vi "FID Scan.vi"(6 "Purpose":string, 8 "error in (no error)":errorcluster) -> (0 "error out":errorcluster, 1 "Cancel ?":bool, 3 "data":T1)   [LabVIEW 2020]
uses:
  Controls/1775E_Authen_Level.ctl
  Controls/user_log.ctl
  <vilib>/Utility/miscctls.llb/LVPointTypeDef.ctl
  Controls/User_DB.ctl
  <vilib>/Instr/_visa.llb/VISA Configure Serial Port (Instr).vi
  <vilib>/addons/database/Connection.llb/Conn Execute.vi
  <vilib>/addons/database/Recordset.llb/Rec Fetch Recordset Data (R).vi
  691E_Global.vi
  <vilib>/addons/database/Recordset.llb/Rec Destroy - Connection.vi
  <vilib>/addons/database/NI_Database_API.lvlib
panel:
  out "Cmd Suceed?":bool
  in  "Hide":bool
  out "Device Info":string
  out "Array":string[](array[string])
  out "State":string
  out "Numeric":i32
  in  "Password":string
  in  "Cancel":bool
  in  "Ok":bool
  in  "View Log":bool
  out "Cmd.":bool
  in  "Super User":bool
  in  "View All":bool
  out "String":string
  in  "Clock No.":string(combo)
  in  "Level":T2
  in  "User Name":string(combo)
  in  "ID Number":i16
  out "Finger Present?":bool
  out "Response":string
  in  "Delete All":bool
  in  "Delete":bool
  in  "Search":bool
  in  "Enroll":bool
  out "Status":string
  out "elements":u8[](array[numeric]) format="%.0x"
  in  "Stop":bool
  out "Buffer Out":string
  in  "write buffer":string="ï\u0001ÿÿÿÿ\u0001\u0000\u00034\u00008"
  out "Profile Image":picture
  # "User Access Login"
  # "thumb finger"
  # "EF01 FFFF FFFF 0700 0700 0003 00A4 00B5"
  # "EF01 FFFF FFFF 0700 0709 0003 0028 0042"
  # "EF01 FFFF FFFF 0700 0700 0000 0065 0073"
  # "EF01 FFFF FFFF 0700 0700 0001 0084 0093"
  # "EF01 FFFF FFFF 0700 0709 0003 0002 001C"
  # "wrong finger"
  # "EF01 FFFF FFFF 0700 0703 0000 0000 0011"
  # "NO finger"
  # "EF01 FFFF FFFF 0700 0703 0000 0000 0011"
  # "EF01 FFFF FFFF 0700 0703 0000 0000 0011"
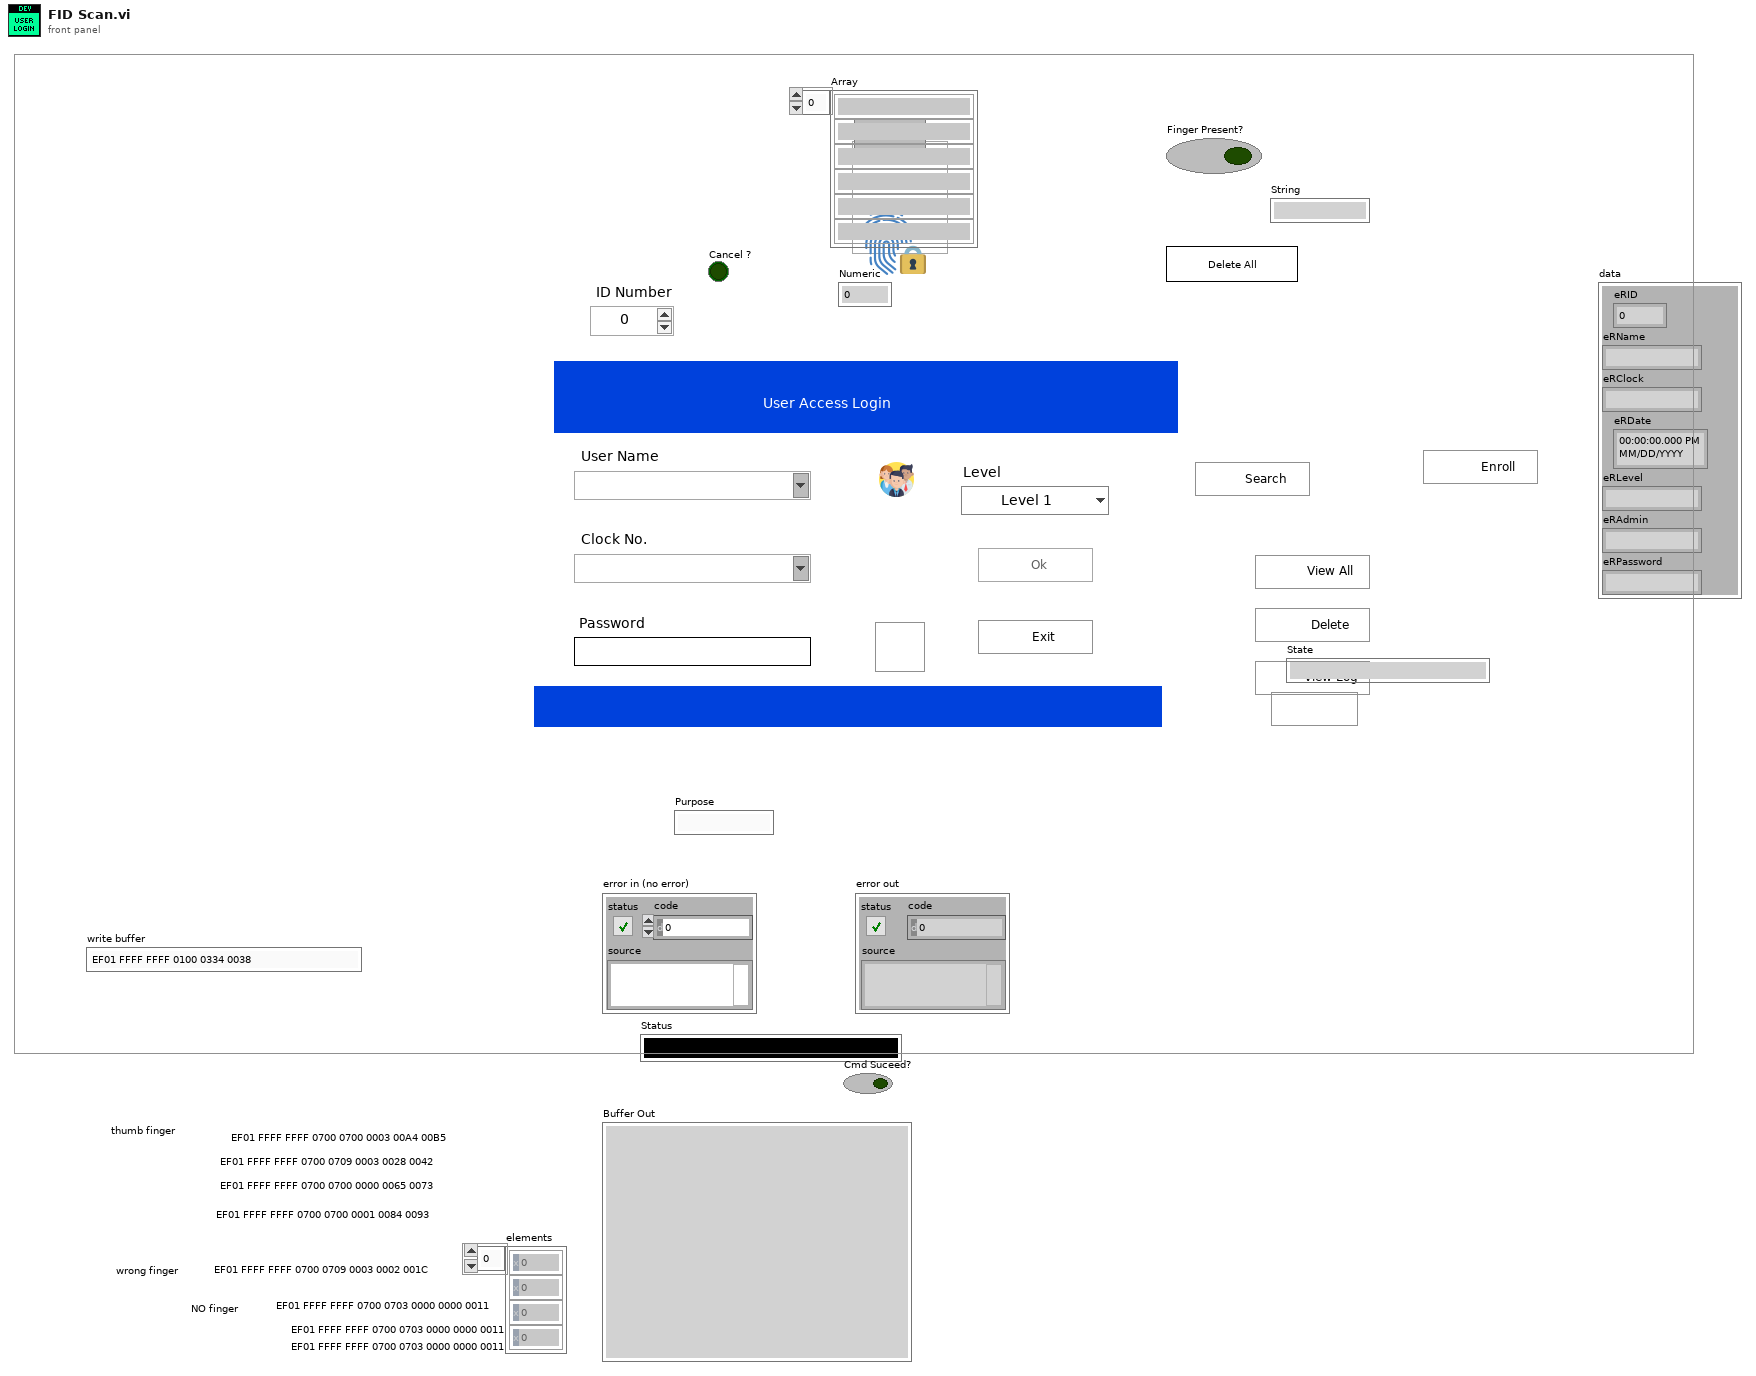
[diagram p1: front panel]
types:
  T1 = typedef "user_log.ctl" = cluster{"eRID":u16, "eRName":string, "eRClock":string, "eRDate":timestamp, "eRLevel":string, "eRAdmin":string, "eRPassword":string}
  T2 = typedef "1775E_Authen_Level.ctl" = enum16{"Level 1", "Level 2", "Level 3", "Level 4", "Super Level"}
  T3 = typedef "LVPointTypeDef.ctl" = cluster{"Horizontal":i16, "Vertical":i16}
  T4 = enum8{"Enabled", "Disabled", "Disabled and Grayed Out"}
  T5 = typedef "TD SQL.ctl" = cluster{"MS SQL Connection":T6, "UDL File":path, "Time":string, "DCODE":string, "WIP+1":i64, "MC No?":i32, "POKAYOKE?":bool, "Expected Result":string, "Result [Status]":string, "Clock":dbl, "RFID":string, "WIP Queue":refnum<queue>, "TS Parameter":T7, "Data_Queue":refnum<queue>[], "RFID Serial No.":string}
  T6 = typedef "NI_Database_API.lvlib/Conn ObjectReference.ctl" = refnum<k1>
  T7 = typedef "TS_Parameter.ctl" = cluster{"ProfitCenterCode":string, "LineCode":string, "WorkOrderNumber":string, "Model":string, "Model_with_Prefix":string, "VendorCode":string, "SetParameterDateCode":string, "PokaYoke":i32, "Target":i32, "Live_DateCode":string, "CustomerPartNumber":string, "Hand":string, "sBarcode":bool, "FCA":i32, "Ent_Stamp":timestamp, "STS_CD":dbl}
  T8 = typedef "User_DB.ctl" = cluster{"eRID":u16, "eRName":string, "eRClock":string, "eRDate":timestamp, "eRLevel":string, "eRAdmin":string, "eRPassword":string, "eRPurpose":string}
  T9 = typedef "NI_Database_API.lvlib/Rec ObjectReference.ctl" = refnum<k1>
  T10 = typedef "LVBoundsTypeDef.ctl" = cluster{"Width":u32, "Height":u32}
  T11 = typedef "imagedata.ctl" = cluster{"image type":i32, "image depth":i32, "image":u8[], "mask":u8[], "colors":u32[], "Rectangle":cluster{"left":i16, "top":i16, "right":i16, "bottom":i16}}
  T12 = cluster{"left":i16, "top":i16, "right":i16, "bottom":i16}
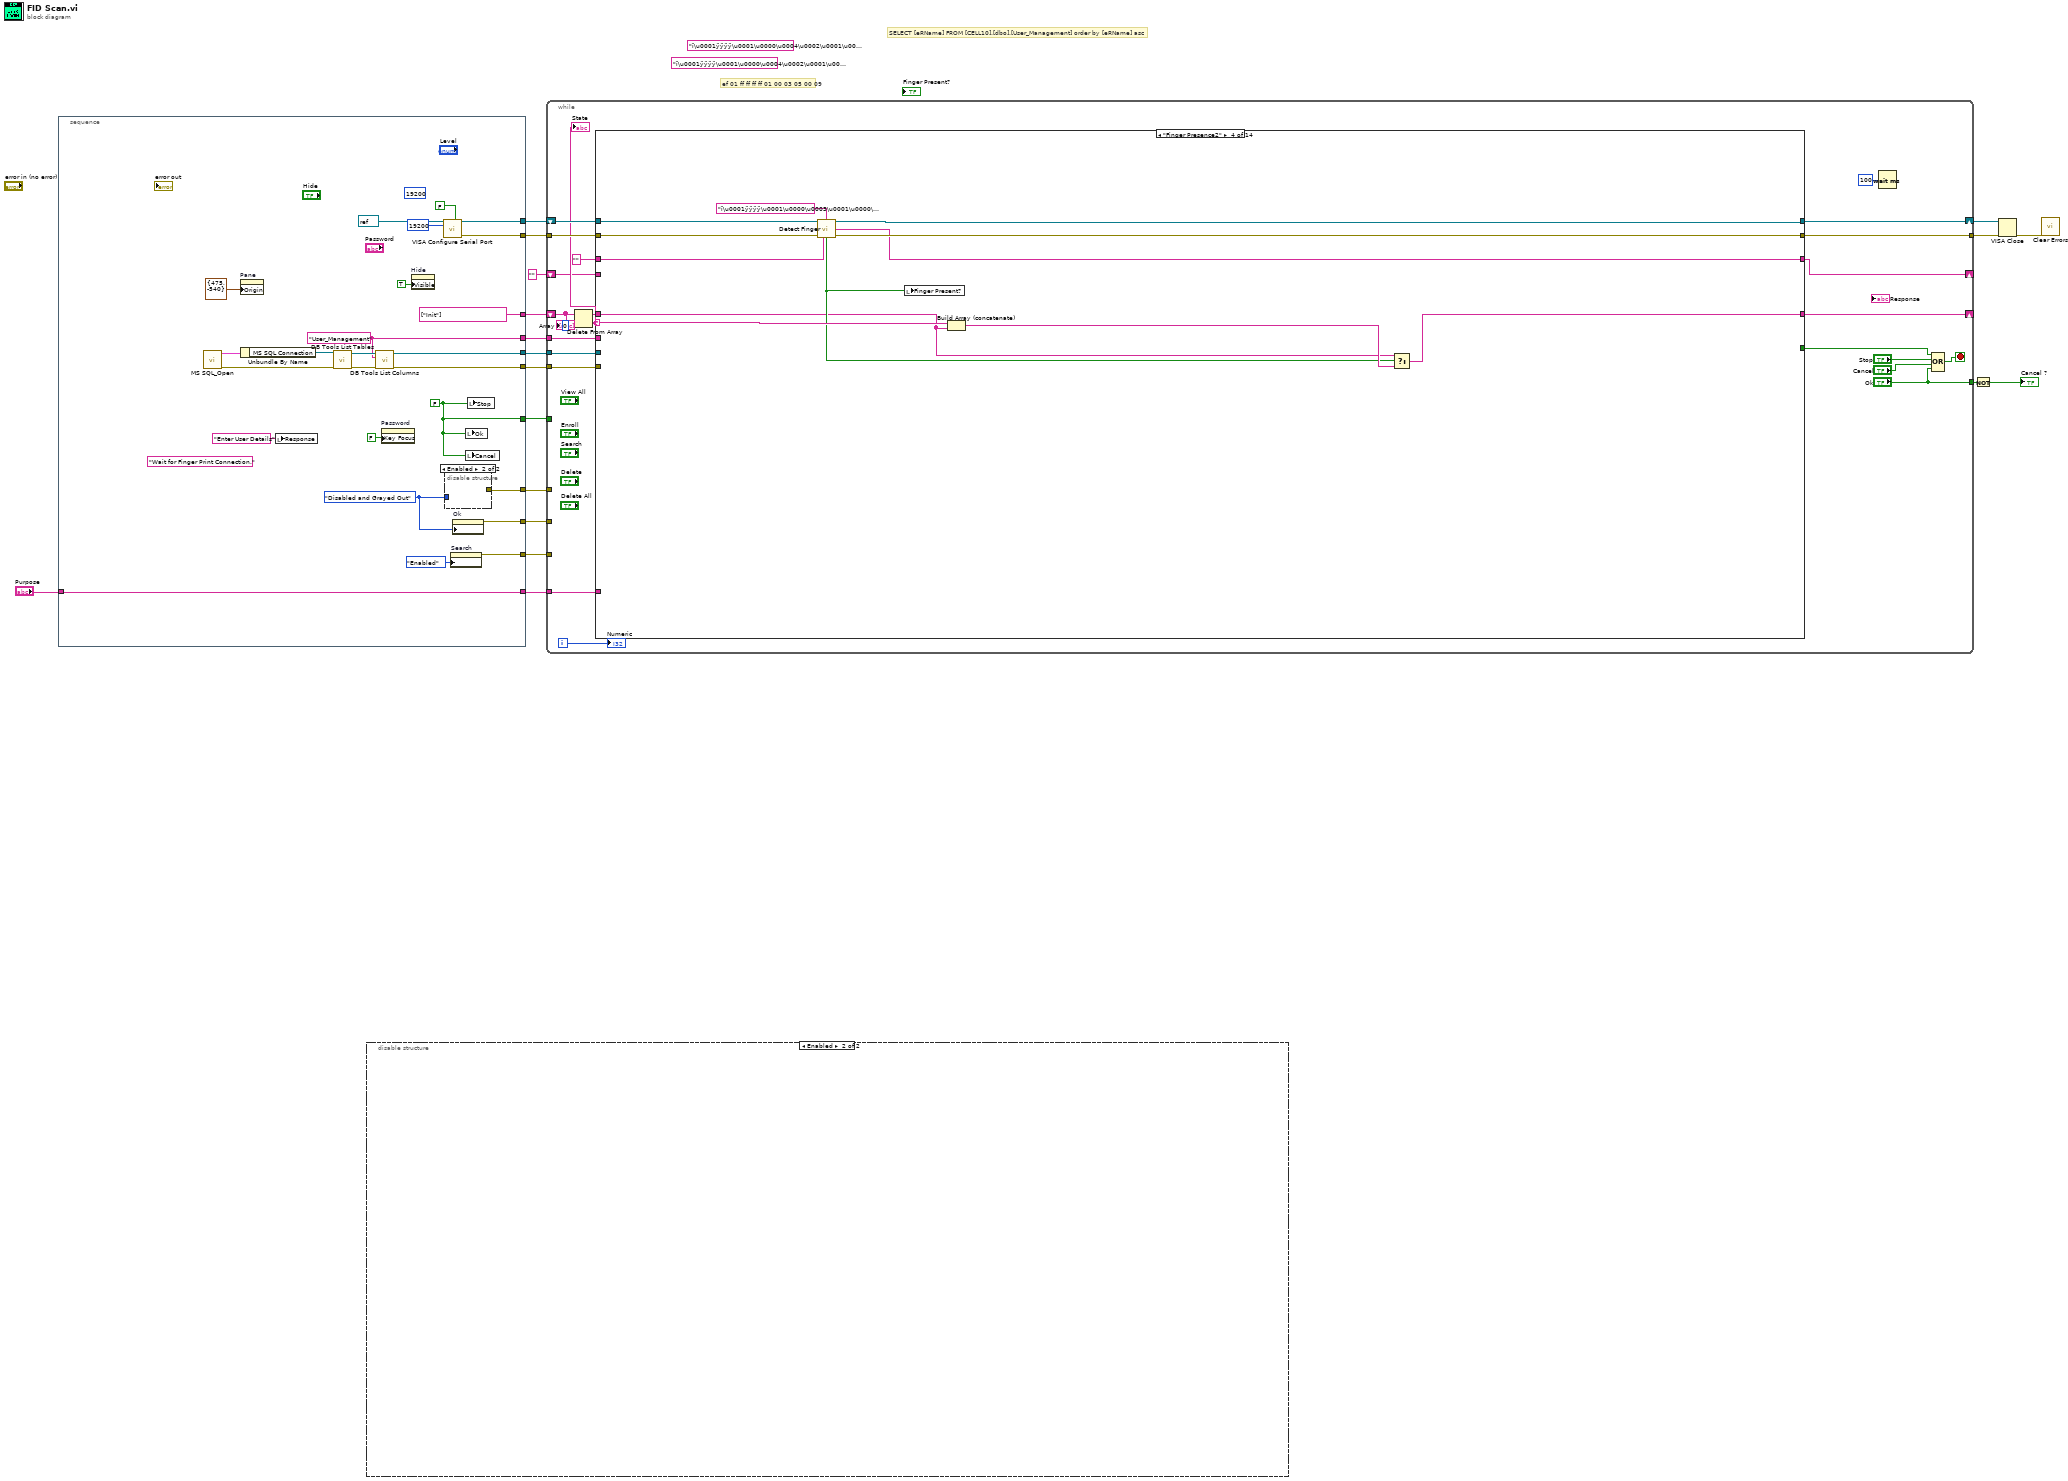
[diagram p0: block diagram]
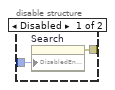
[diagram p2: hidden frame]
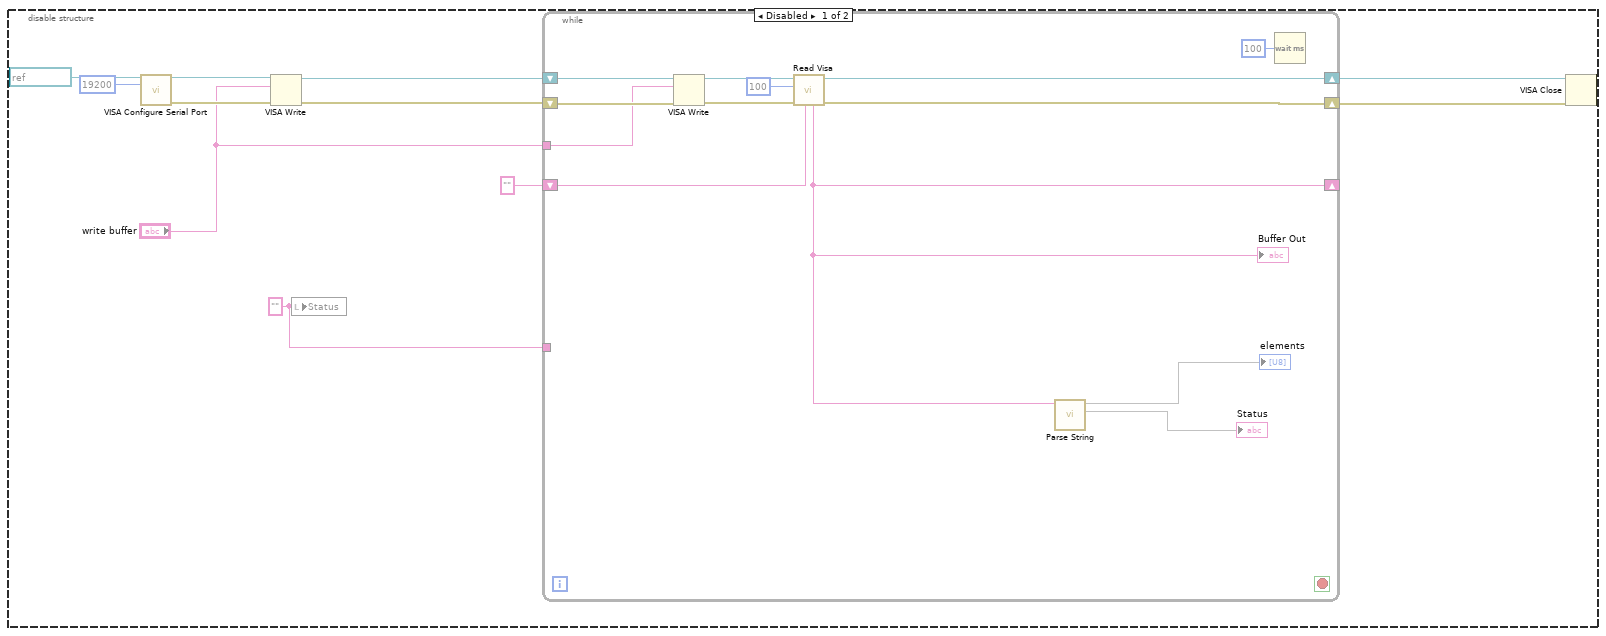
[diagram p3: hidden frame]
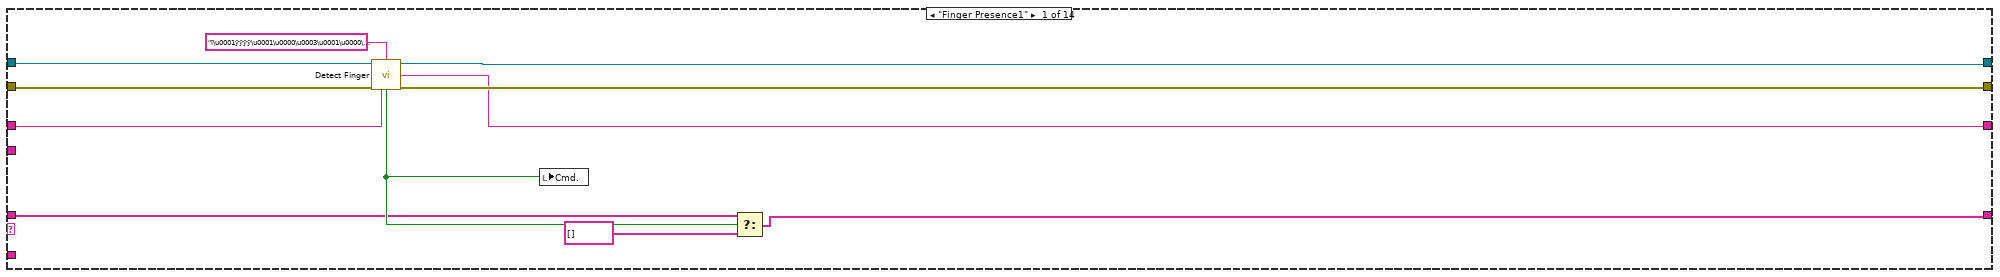
[diagram p4: hidden frame]
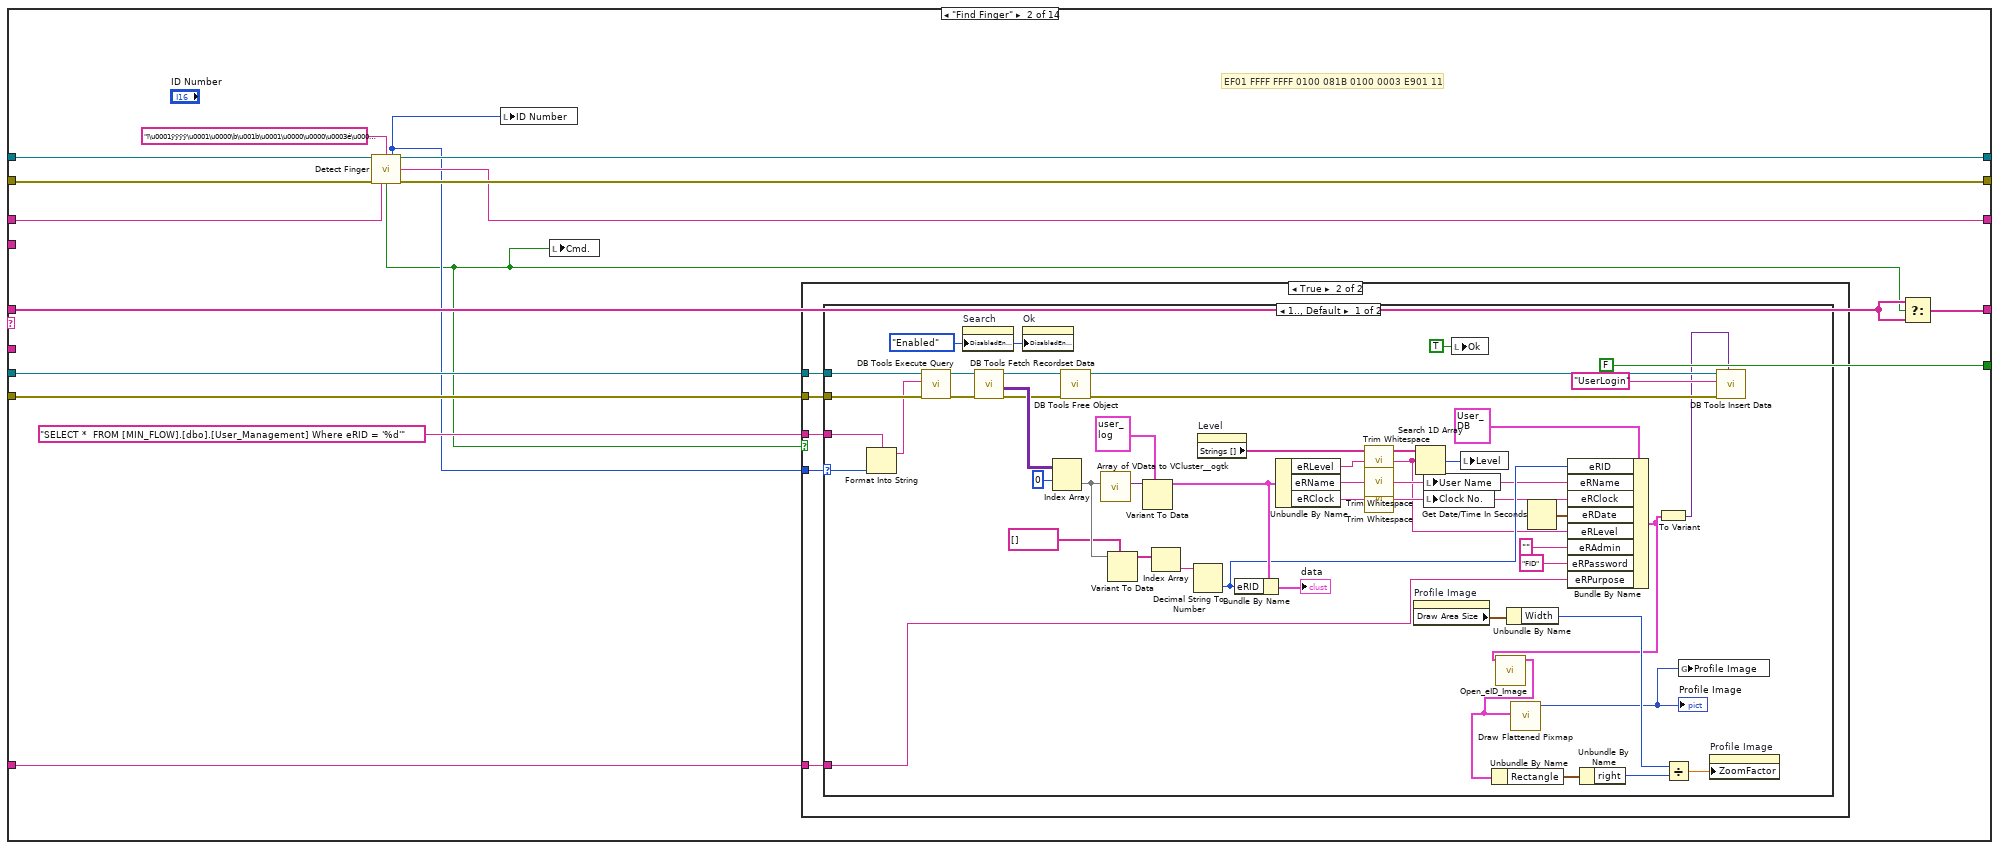
[diagram p5: hidden frame]
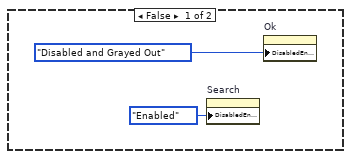
[diagram p6: hidden frame]
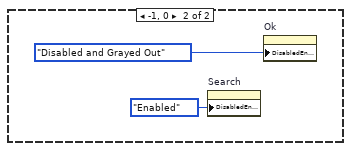
[diagram p7: hidden frame]
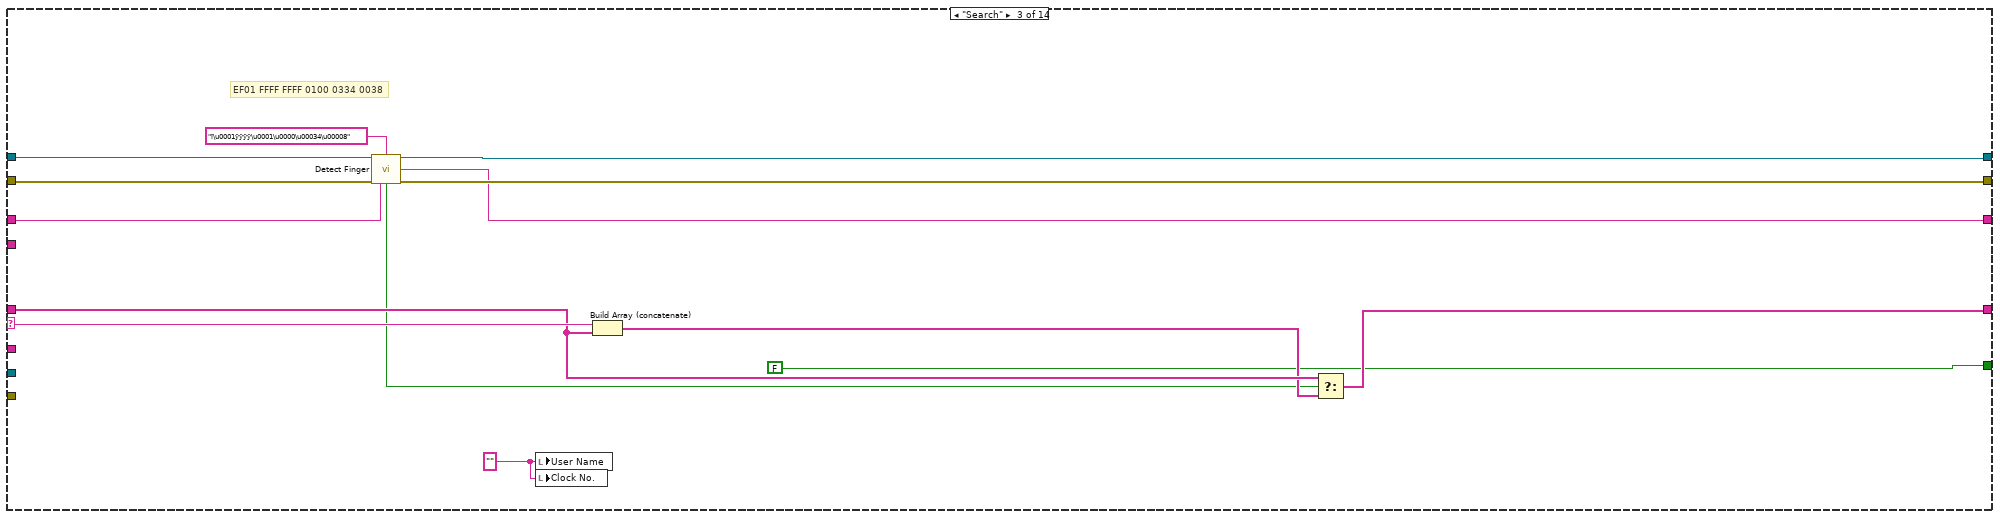
[diagram p8: hidden frame]
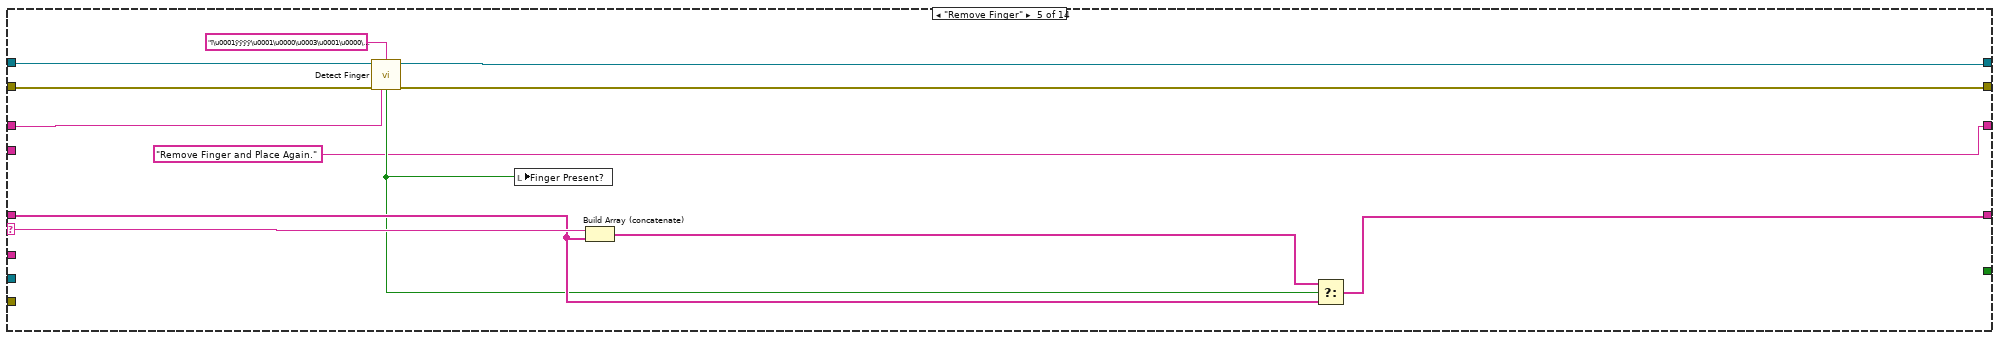
[diagram p9: hidden frame]
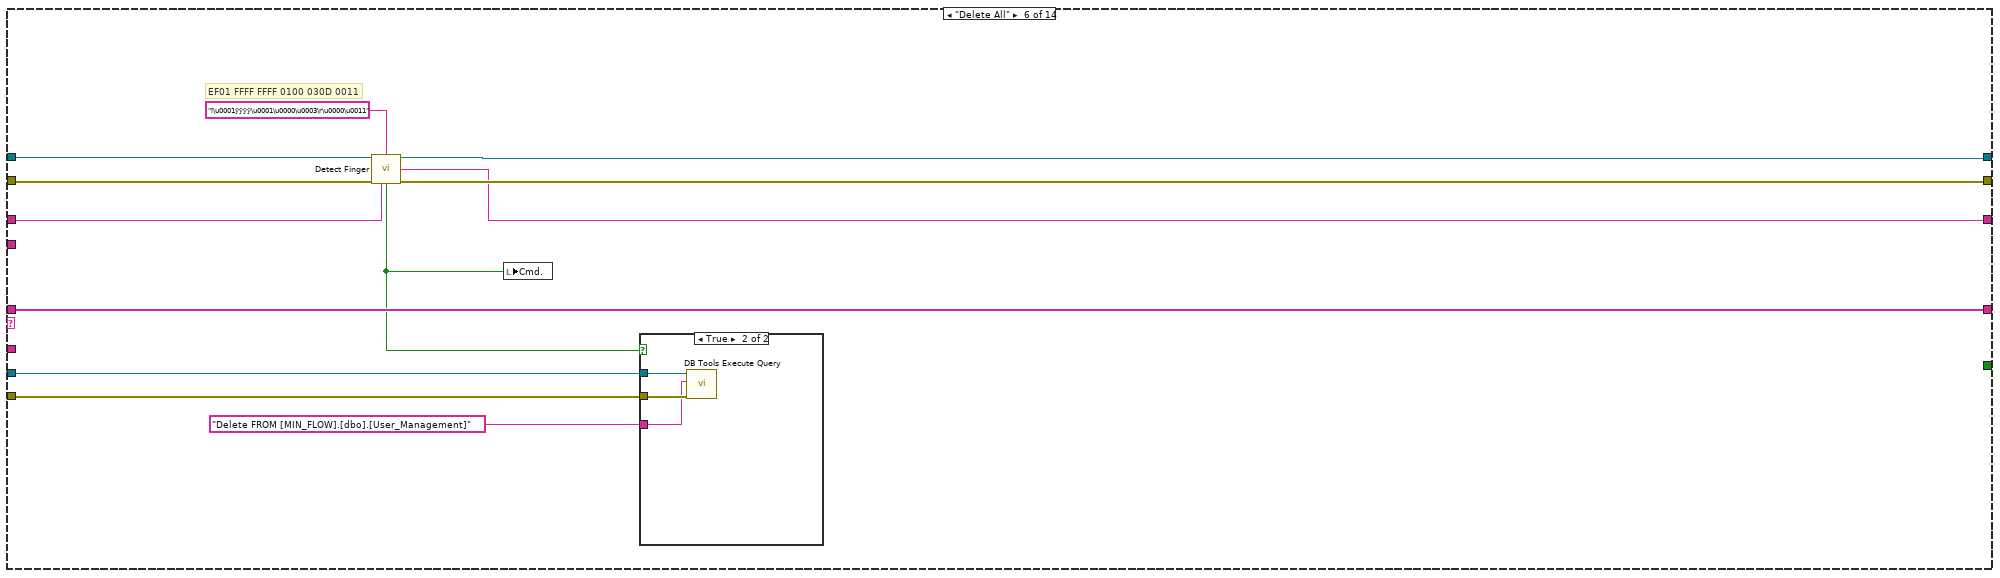
[diagram p10: hidden frame]
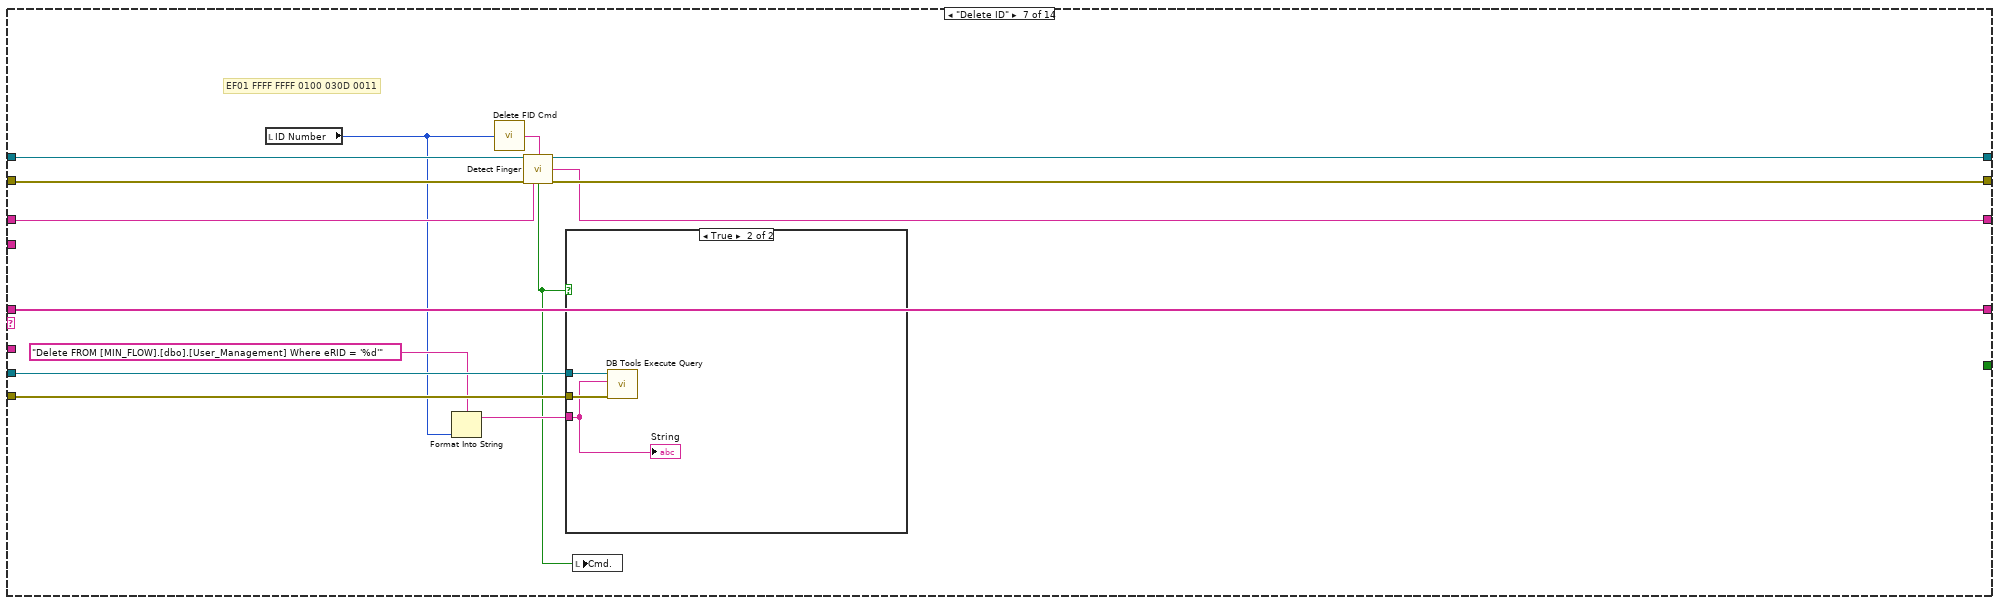
[diagram p12: hidden frame]
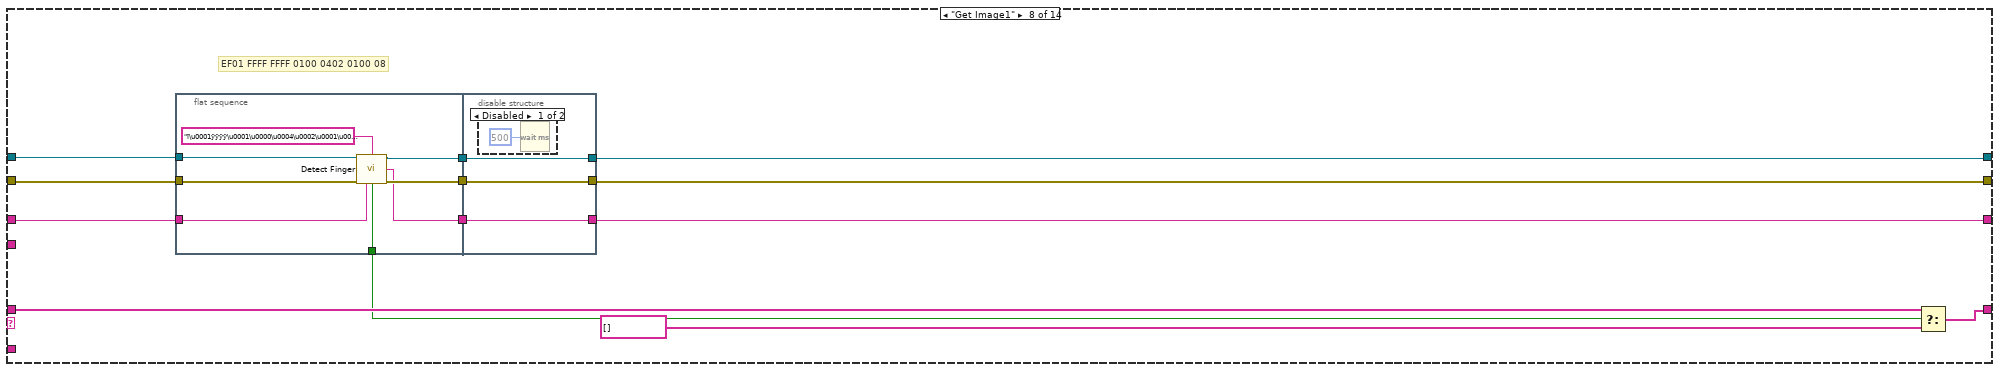
[diagram p14: hidden frame]
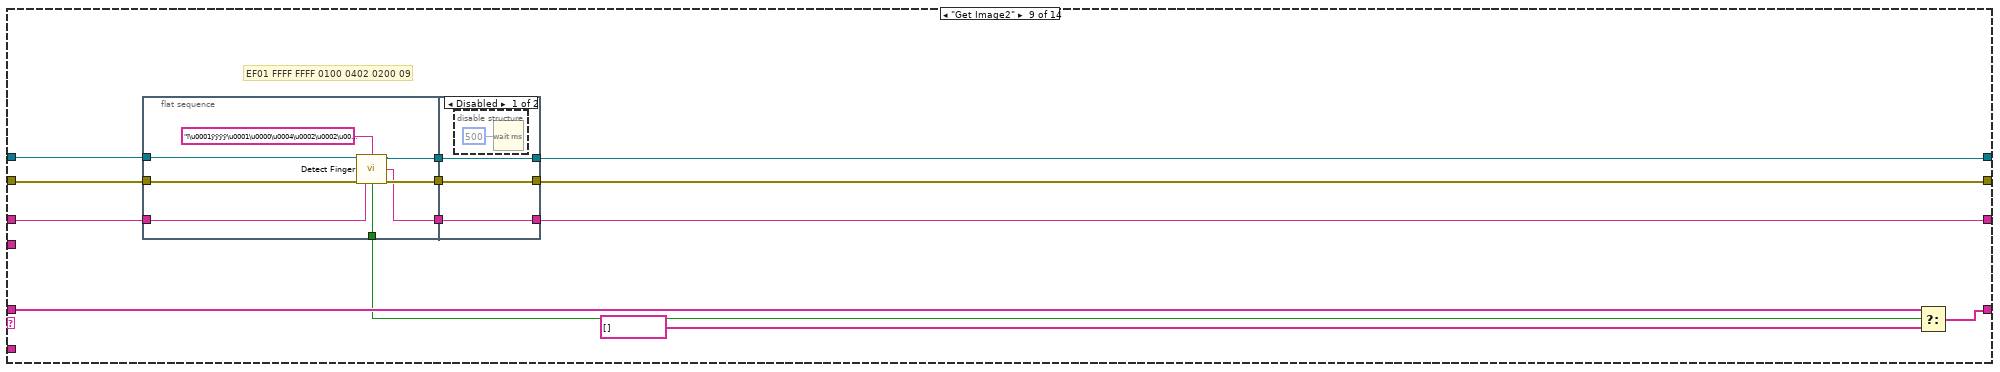
[diagram p16: hidden frame]
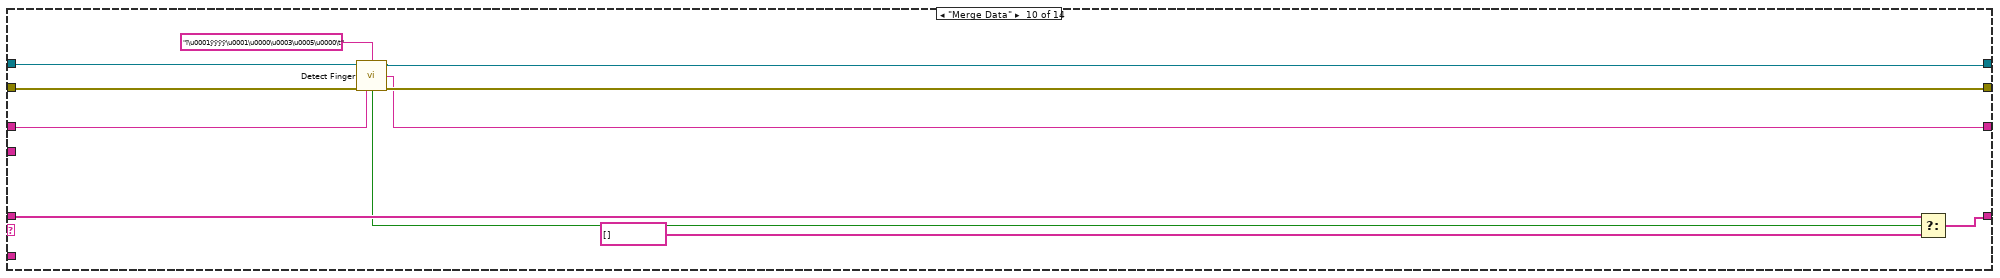
[diagram p18: hidden frame]
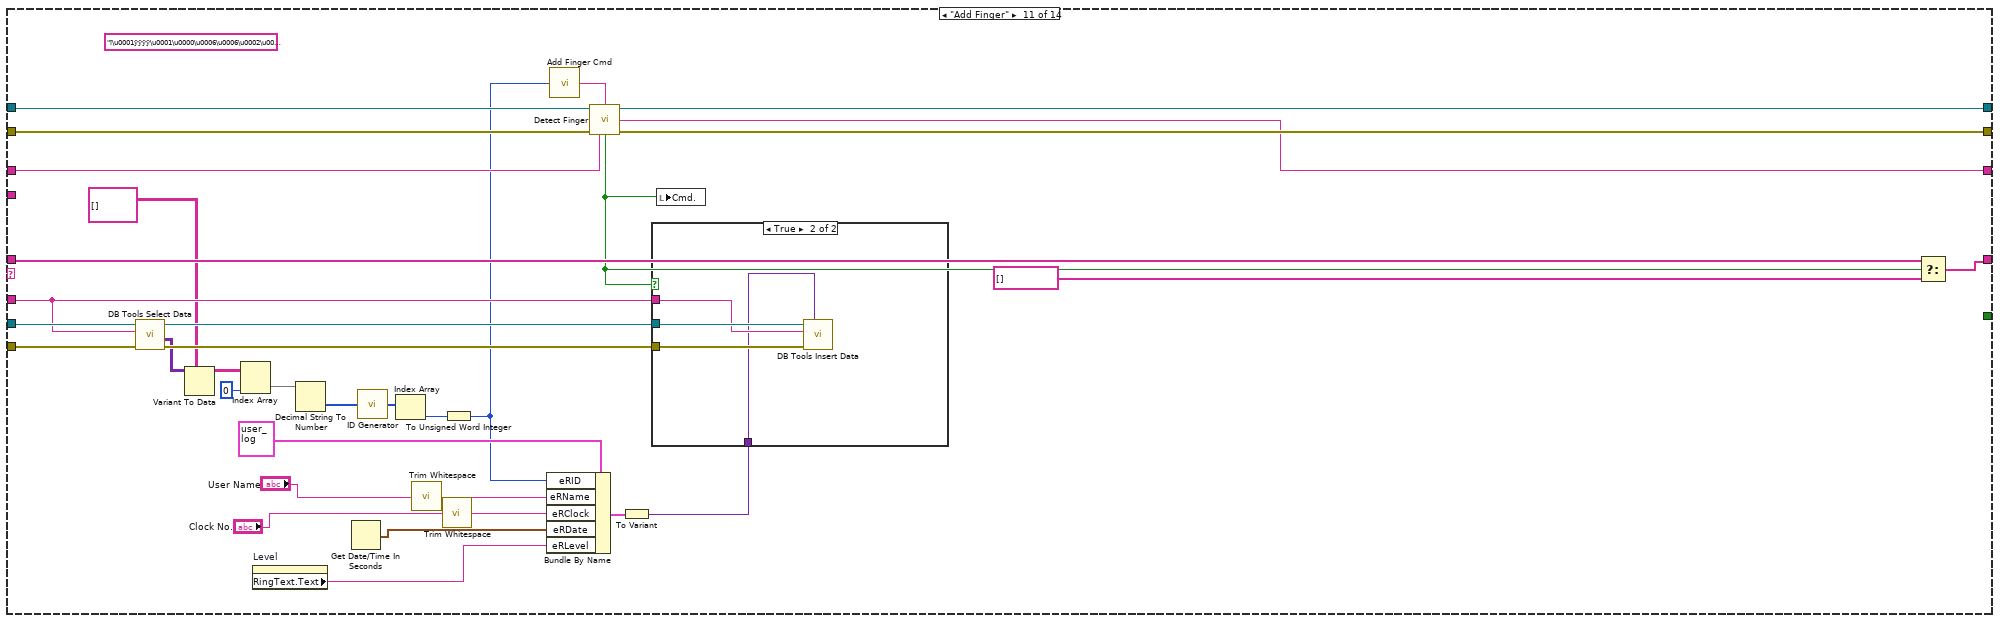
[diagram p19: hidden frame]
diagram:
  (unwired) "ï\u0001ÿÿÿÿ\u0001\u0000\u0004\u0002\u0001\u0000\b" ("write buffer")
  (unwired) "ï\u0001ÿÿÿÿ\u0001\u0000\u0004\u0002\u0001\u0000\b" ("write buffer")
  # "SELECT [eRName] FROM [CELL10].[dbo].[User_Management] order by [eRName] asc"
  # "ef 01 ff ff ff ff 01 00 03 05 00 09"
  n1 = stacked-sequence {
    tunnel: [string[] ["Init"]] -> w18
    tunnel: [w41] -> w17
    tunnel: [w40] -> w16
    tunnel: [w37] -> w11
    tunnel: [w36] -> w10
    tunnel: [w35] -> w9
    tunnel: [w34] -> w6
    tunnel: [w32] -> w5
    tunnel: [w31] -> w4
    tunnel: [w29] -> w3
    tunnel: [w20] -> w2
    tunnel: "Purpose" -> [w20]
    frame #0 {
      (unwired) "Wait for Finger Print Connection." ("Response")
      (unwired) u32 19200 ("baud rate (9600)")
      w33 = T4."Disabled and Grayed Out" ("Disabled")
      w34 = FALSE ("Stop")
      w35 = "User_Management" ("table")
      n2 = call "MS SQL_Open.vi"() -> ("error out"=w21:errorcluster, "Ref Out"=w23:T5)  [unwired: 9 in, 1 out]
      n3 = property on="Pane" class="Pane"("Origin"=T3 {"Horizontal"=475, "Vertical"=-540}) -> ()  [unwired: 2 in, 2 out]
      n4 = Unbundle By Name(w23) -> ("MS SQL Connection"=w22:T6)
      n5 = local write "Response"("Enter User Details" ("Response")) -> ()
      n6 = call <vilib>:"DB Tools List Tables.vi"("error in (no error)"=w21, "connection reference"=w22) -> ("error out"=w38:errorcluster, "connection reference out"=w39:T6)  [unwired: 3 in, 1 out]
      n7 = call <vilib>:"DB Tools List Columns.vi"("error in (no error)"=w38, "table"=w35, "connection reference"=w39) -> ("error out"=w36:errorcluster, "connection reference out"=w37:T6)  [unwired: 1 in, 2 out]
      n8 = property on="Password" class="Str"("Key Focus"=FALSE) -> ()  [unwired: 2 in, 2 out]
      n9 = property on="Hide" class="Bool"("Visible"=TRUE) -> ()  [unwired: 2 in, 2 out]
      n10 = call-poly "VISA Configure Serial Port"("VISA resource name"=refnum<visa-resource-name> refnum ("FID_Comm"), "Enable Termination\nChar (T)"=FALSE ("Enable Termination\nChar (T)"), "baud rate (9600)"=u32 19200) -> ("VISA resource name out"=w41:refnum<visa-resource-name>, "error out"=w40:errorcluster)  [unwired: 11 in]
      n11 = disable-structure shown="Enabled" {
        disable-tunnel: w33 -> [w45 _]
        disable-tunnel: [w44 _] -> w32
        frame Disabled {
          n12 = property on="Search" class="Bool (strict)"("DisabledEnum"=w45) -> (error out=w44:errorcluster)  [unwired: 2 in, 1 out]
        }
        frame Enabled {
        }
      }
      n13 = property on="Search" class="Bool (strict)"("DisabledEnum"=T4."Enabled" ("Disabled")) -> (error out=w29:errorcluster)  [unwired: 2 in, 1 out]
      n14 = property on="Ok" class="Bool (strict)"("DisabledEnum"=w33) -> (error out=w31:errorcluster)  [unwired: 2 in, 1 out]
      n15 = local write "Ok"(w34) -> ()
      n16 = local write "Cancel"(w34) -> ()
      n17 = local write "Stop"(w34) -> ()
    }
  }
  n18 = disable-structure shown="Enabled" {
    frame Disabled {
      w46 = "" ("Status")
      n19 = call-poly "VISA Configure Serial Port"("VISA resource name"=refnum<visa-resource-name> "COM6", "baud rate (9600)"=u32 19200) -> ("VISA resource name out"=w52:refnum<visa-resource-name>, "error out"=w50:errorcluster)  [unwired: 12 in]
      n20 = VISA Write(VISA resource name=w52, write buffer="write buffer", error in (no error)=w50) -> (VISA resource name out=w51:refnum<visa-resource-name>, error out=w49:errorcluster)  [unwired: 1 out]
      n21 = local write "Status"(w46) -> ()
      n22 = while {
        shift-right: [w70] -> w54
        shift-left: w51 -> [w64]
        shift-right: [w69] -> w53
        shift-left: w49 -> [w63]
        shift-right: [w59] -> _
        shift-left: "" ("Buffer Out") -> [w65]
        tunnel: "write buffer" -> [w60]
        tunnel: w46 -> [_]
        stop <- w67 stop-if-true
        n23 = VISA Write(VISA resource name=w64, write buffer=w60, error in (no error)=w63) -> (VISA resource name out=w61:refnum<visa-resource-name>, error out=w62:errorcluster)  [unwired: 1 out]
        n24 = call <userlib>:"Read Visa.vi"("Buffer In"=w65, "error in (no error)"=w62, "delay before read (ms)"=u32 100, "VISA Refnum in"=w61) -> ("error out"=w69:errorcluster, "VISA Refnum out"=w70:refnum<visa-resource-name>, "Buffer Out"=w59:string)  [unwired: 5 in]
        "Buffer Out" <- w59
        n25 = call "Parse String.vi"("Ack package"=w59) -> (2:→"Status", 3:→"elements")  [unwired: 7 in, 2 out]
        n26 = Wait (ms)(milliseconds to wait=u32 100) -> ()  [unwired: 1 out]
      }
      n27 = VISA Close(VISA resource name=w54, error in (no error)=w53) -> ()  [unwired: 1 out]
    }
    frame Enabled {
    }
  }
  n28 = while {
    shift-right: [w92] -> _
    shift-left: w18 -> [w93]
    tunnel: w16 -> [w90]
    shift-right: [w89] -> w14
    shift-left: w17 -> [w91]
    shift-right: [w79] -> _
    shift-left: "" ("Buffer Out") -> [w80]
    tunnel: [w86] -> w13
    tunnel: w11 -> [w78]
    tunnel: w10 -> [w77]
    tunnel: w9 -> [w76]
    tunnel: w6 -> [_]
    tunnel: ["Ok"] -> w8
    tunnel: w5 -> [_]
    tunnel: w4 -> [_]
    tunnel: w3 -> [_]
    tunnel: w2 -> [w71]
    i -> [w73]
    stop <- w84 stop-if-true
    n29 = Delete From Array(array=w93, index=0) -> (deleted portion=w83:string, array with subset deleted=w87:string[])  [unwired: 1 in]
    "State" <- w83
    n30 = case shown="\"Finger Presence2\"" w83 {
      selector: w83 -> [_ _ w190 w202 w214 _ _ _ _ _ _ _ _ _]
      tunnel: w87 -> [w95 w111 w189 w192 w213 w219 w236 w259 w284 w307 w341 w346 w360 w646]
      tunnel: [w94 w120 w187 w191 w211 w219 w236 w258 w283 w306 w340 w346 w359 w646] -> w92
      tunnel: w91 -> [w104 w119 w186 w200 w210 w226 w243 w256 w281 w304 w338 w349 w358 w644]
      tunnel: w90 -> [w103 w118 w185 w199 w209 w225 w242 w255 w280 w303 w337 w348 w357 w641]
      tunnel: [w101 w116 w183 w197 w207 w223 w240 w254 w279 w302 w336 w349 w356 w643] -> w89
      tunnel: [w102 w117 w184 w198 w208 w224 w241 w253 w278 w301 w335 w348 w355 w640] -> w86
      tunnel: [w100 w115 w182 w196 "Remove Finger and Place Again." ("Response") w222 w239 w251 w276 w299 w334 w347 w354 w645] -> w79
      tunnel: "" ("Buffer Out") -> [w97 w113 w178 w193 w204 w220 w238 w247 w272 w297 w332 w347 _ w642]
      tunnel: [_ FALSE ("Stop") FALSE ("Stop") _ _ _ _ _ _ _ _ _ _ _] -> w82
      tunnel: w80 -> [_ _ _ _ _ _ _ _ _ _ _ _ w354 _]
      tunnel: w78 -> [_ w110 _ _ _ w218 w235 _ _ _ w331 _ w353 w636]
      tunnel: w77 -> [_ w109 _ _ _ w217 w234 _ _ _ w330 _ w352 _]
      tunnel: w76 -> [_ _ _ _ _ _ _ _ _ _ w326 _ w351 _]
      tunnel: w71 -> [_ w105 _ _ _ _ _ _ _ _ _ _ w350 _]
      frame "Finger Presence1" {
        n31 = call "Detect Finger.vi"("VISA Refnum in"=w104, "Cmd"="ï\u0001ÿÿÿÿ\u0001\u0000\u0003\u0001\u0000\u0005" ("write buffer"), "error in (no error)"=w103, "Buffer In"=w97) -> ("VISA Refnum out"=w101:refnum<visa-resource-name>, "Response"=w100:string, "Cmd Suceed?"=w98:bool, "error out"=w102:errorcluster)  [unwired: 6 in, 2 out]
        n32 = local write "Cmd."(w98) -> ()
        n33 = Select(t=w95, s=w98, f=string[] []) -> (s? t:f=w94:string[])
      }
      frame "Find Finger" {
        # "EF01 FFFF FFFF 0100 081B 0100 0003 E901 11"
        n34 = call "Detect Finger.vi"("VISA Refnum in"=w119, "Cmd"="ï\u0001ÿÿÿÿ\u0001\u0000\b\u001b\u0001\u0000\u0000\u0003é\u0001\u0011" ("write buffer"), "error in (no error)"=w118, "Buffer In"=w113) -> ("ID"=w107:i16, "VISA Refnum out"=w116:refnum<visa-resource-name>, "Response"=w115:string, "Cmd Suceed?"=w106:bool, "error out"=w117:errorcluster)  [unwired: 6 in, 1 out]
        n35 = local write "ID Number"(w107) -> ()
        n36 = local write "Cmd."(w106) -> ()
        n37 = case shown="True" w106 {
          tunnel: w110 -> [_ w127]
          tunnel: w109 -> [_ w126]
          tunnel: "SELECT *  FROM [MIN_FLOW].[dbo].[User_Management] Where eRID = '%d'" ("SQL query") -> [_ w125]
          tunnel: w107 -> [_ w124]
          tunnel: w105 -> [_ w123]
          frame False {
            n38 = property on="Search" class="Bool (strict)"("DisabledEnum"=T4."Enabled" ("Disabled")) -> ()  [unwired: 2 in, 2 out]
            n39 = property on="Ok" class="Bool (strict)"("DisabledEnum"=T4."Disabled and Grayed Out" ("Disabled")) -> ()  [unwired: 2 in, 2 out]
          }
          frame True {
            n40 = case shown="1.., Default" w124 {
              selector: w124 -> [w171 _]
              tunnel: w127 -> [w153 _]
              tunnel: w126 -> [w173 _]
              tunnel: w125 -> [w172 _]
              tunnel: w123 -> [w128 _]
              frame 1.., Default {
                w140 = T4."Enabled" ("Disabled")
                n41 = Format Into String(format string=w172, w171) -> (resulting string=w170:string)  [unwired: 2 in, 1 out]
                n42 = call-poly <vilib>:"DB Tools Execute Query.vi"("error in (no error)"=w173, "SQL query"=w170, "connection reference"=w153) -> ("error out"=w174:errorcluster, "recordset reference"=w154:T9)  [unwired: 5 in]
                n43 = property on="Search" class="Bool (strict)"("DisabledEnum"=w140) -> ()  [unwired: 2 in, 2 out]
                n44 = call-poly <vilib>:"DB Tools Fetch Recordset Data.vi"("error in (no error)"=w174, "recordset reference"=w154) -> ("error out"=w150:errorcluster, "recordset data"=w166:variant[][], "recordset reference out"=w152:T9)  [unwired: 3 in]
                n45 = property on="Ok" class="Bool (strict)"("DisabledEnum"=w140) -> ()  [unwired: 2 in, 2 out]
                n46 = Index Array(array=w166, index (row)=0 ("disabled index (col)")) -> (element=w165:variant[])  [unwired: 1 in]
                n47 = call-poly <vilib>:"DB Tools Free Object.vi"("error in (no error)"=w150, "recordset reference"=w152) -> ("error out"=w149:errorcluster, "connection reference"=w151:T6)  [unwired: 8 in]
                n48 = call <userlib>:"Array of VData to VCluster__ogtk.vi"("Array"=w165) -> ("VCluster"=w168:variant)  [unwired: 9 in, 1 out]
                n49 = Variant To Data(type=string[] [], Variant=w165) -> (data=w163:string[])  [unwired: 1 in, 1 out]
                n50 = Variant To Data(type=T1 {"eRID"=0, "eRName"="", "eRClock"="", "eRDate"=timestamp(0 s since 1904-01-01), "eRLevel"="", "eRAdmin"="", "eRPassword"=""} ("Cluster"), Variant=w168) -> (data=w160:T1)  [unwired: 1 in, 1 out]
                n51 = Index Array(array=w163) -> (element=w162:string)  [unwired: 1 in]
                n52 = Decimal String To Number(string=w162) -> (number=w146:i32)  [unwired: 2 in, 1 out]
                n53 = property on="Level" class="Enum (strict)"() -> ("Strings []"=w155:string[])  [unwired: 2 in, 2 out]
                n54 = Bundle By Name(cluster=w160, "eRID"=w146) -> (→"data":T1)
                n55 = Unbundle By Name(w160) -> ("eRLevel"=w159:string, "eRName"=w157:string, "eRClock"=w156:string)
                n56 = call <vilib>:"Trim Whitespace.vi"("string"=w159) -> ("trimmed string"=w143:string)  [unwired: 1 in]
                n57 = call <vilib>:"Trim Whitespace.vi"("string"=w157) -> ("trimmed string"=w145:string)  [unwired: 1 in]
                n58 = call <vilib>:"Trim Whitespace.vi"("string"=w156) -> ("trimmed string"=w144:string)  [unwired: 1 in]
                n59 = property on="Profile Image" class="Pict"() -> ("Draw Area Size"=w133:T10)  [unwired: 2 in, 2 out]
                n60 = Search 1D Array(1D array=w155, element=w143) -> (index of element=w158:i32)  [unwired: 1 in]
                n61 = local write "User Name"(w145) -> ()
                n62 = local write "Clock No."(w144) -> ()
                n63 = local write "Ok"(TRUE ("Ok")) -> ()
                n64 = local write "Level"(w158) -> ()
                n65 = Unbundle By Name(w133) -> ("Width"=w135:u32)
                n66 = Get Date/Time In Seconds() -> (seconds since 1Jan1904=w142:timestamp)
                n67 = Bundle By Name(cluster=T8 {"eRID"=0, "eRName"="", "eRClock"="", "eRDate"=timestamp(0 s since 1904-01-01), "eRLevel"="", "eRAdmin"="", "eRPassword"="", "eRPurpose"=""} ("Cluster"), "eRID"=w146, "eRName"=w145, "eRClock"=w144, "eRDate"=w142, "eRLevel"=w143, "eRAdmin"="", "eRPassword"="FID", "eRPurpose"=w128) -> (w131:T8)
                n68 = call "Open_eID_Image.vi"("eID"=w131) -> ("image data"=w130:T11)  [unwired: 10 in]
                n69 = Unbundle By Name(w130) -> ("Rectangle"=w132:T12)
                n70 = call <vilib>:"Draw Flattened Pixmap.vi"("image data"=w130) -> ("new picture"=w129:picture)  [unwired: 8 in]
                "Profile Image" <- w129
                n71 = Unbundle By Name(w132) -> ("right"=w134:i16)
                n72 = To Variant(anything=w131) -> (Variant=w141:variant)
                n73 = Divide(x=w135, y=w134) -> (x/y=w136:dbl)
                n74 = global write "691E_Global.vi" "Profile Image"(w129) -> ()
                n75 = property on="Profile Image" class="Pict"("ZoomFactor"=w136) -> ()  [unwired: 2 in, 2 out]
                n76 = call <vilib>:"DB Tools Insert Data.vi"("data"=w141, "error in (no error)"=w149, "table"="UserLogin", "connection reference"=w151) -> ()  [unwired: 6 in, 2 out]
              }
              frame -1, 0 {
                n77 = property on="Search" class="Bool (strict)"("DisabledEnum"=T4."Enabled" ("Disabled")) -> ()  [unwired: 2 in, 2 out]
                n78 = property on="Ok" class="Bool (strict)"("DisabledEnum"=T4."Disabled and Grayed Out" ("Disabled")) -> ()  [unwired: 2 in, 2 out]
              }
            }
          }
        }
        n79 = Select(t=w111, s=w106, f=w111) -> (s? t:f=w120:string[])
      }
      frame "Search" {
        w177 = "" ("User Name")
        # "EF01 FFFF FFFF 0100 0334 0038"
        n80 = call "Detect Finger.vi"("VISA Refnum in"=w186, "Cmd"="ï\u0001ÿÿÿÿ\u0001\u0000\u00034\u00008" ("write buffer"), "error in (no error)"=w185, "Buffer In"=w178) -> ("VISA Refnum out"=w183:refnum<visa-resource-name>, "Response"=w182:string, "Cmd Suceed?"=w180:bool, "error out"=w184:errorcluster)  [unwired: 6 in, 2 out]
        n81 = local write "User Name"(w177) -> ()
        n82 = local write "Clock No."(w177) -> ()
        n83 = Build Array (concatenate)(w190, w189) -> (w188:string[])
        n84 = Select(t=w189, s=w180, f=w188) -> (s? t:f=w187:string[])
      }
      frame "Finger Presence2" {
        n85 = call "Detect Finger.vi"("VISA Refnum in"=w200, "Cmd"="ï\u0001ÿÿÿÿ\u0001\u0000\u0003\u0001\u0000\u0005" ("write buffer"), "error in (no error)"=w199, "Buffer In"=w193) -> ("VISA Refnum out"=w197:refnum<visa-resource-name>, "Response"=w196:string, "Cmd Suceed?"=w194:bool, "error out"=w198:errorcluster)  [unwired: 6 in, 2 out]
        n86 = local write "Finger Present?"(w194) -> ()
        n87 = Build Array (concatenate)(w202, w192) -> (w201:string[])
        n88 = Select(t=w192, s=w194, f=w201) -> (s? t:f=w191:string[])
      }
      frame "Remove Finger" {
        n89 = call "Detect Finger.vi"("VISA Refnum in"=w210, "Cmd"="ï\u0001ÿÿÿÿ\u0001\u0000\u0003\u0001\u0000\u0005" ("write buffer"), "error in (no error)"=w209, "Buffer In"=w204) -> ("VISA Refnum out"=w207:refnum<visa-resource-name>, "Cmd Suceed?"=w205:bool, "error out"=w208:errorcluster)  [unwired: 6 in, 3 out]
        n90 = local write "Finger Present?"(w205) -> ()
        n91 = Build Array (concatenate)(w214, w213) -> (w212:string[])
        n92 = Select(t=w212, s=w205, f=w213) -> (s? t:f=w211:string[])
      }
      frame "Delete All" {
        # "EF01 FFFF FFFF 0100 030D 0011"
        n93 = call "Detect Finger.vi"("VISA Refnum in"=w226, "Cmd"="ï\u0001ÿÿÿÿ\u0001\u0000\u0003\r\u0000\u0011" ("write buffer"), "error in (no error)"=w225, "Buffer In"=w220) -> ("VISA Refnum out"=w223:refnum<visa-resource-name>, "Response"=w222:string, "Cmd Suceed?"=w215:bool, "error out"=w224:errorcluster)  [unwired: 6 in, 2 out]
        n94 = local write "Cmd."(w215) -> ()
        n95 = case shown="True" w215 {
          tunnel: w218 -> [_ w229]
          tunnel: w217 -> [_ w228]
          tunnel: "Delete FROM [MIN_FLOW].[dbo].[User_Management]" ("SQL query") -> [_ w227]
          frame False {
          }
          frame True {
            n96 = call-poly <vilib>:"DB Tools Execute Query.vi"("error in (no error)"=w228, "SQL query"=w227, "connection reference"=w229) -> ()  [unwired: 5 in, 2 out]
          }
        }
      }
      frame "Delete ID" {
        # "EF01 FFFF FFFF 0100 030D 0011"
        n97 = local read "ID Number"() -> (w231:i16)
        n98 = Format Into String(format string="Delete FROM [MIN_FLOW].[dbo].[User_Management] Where eRID = '%d'" ("SQL query"), w231) -> (resulting string=w232:string)  [unwired: 2 in, 1 out]
        n99 = call "Delete FID Cmd.vi"("ID"=w231) -> ("Cmd"=w237:string)
        n100 = call "Detect Finger.vi"("VISA Refnum in"=w243, "Cmd"=w237, "error in (no error)"=w242, "Buffer In"=w238) -> ("VISA Refnum out"=w240:refnum<visa-resource-name>, "Response"=w239:string, "Cmd Suceed?"=w230:bool, "error out"=w241:errorcluster)  [unwired: 6 in, 2 out]
        n101 = case shown="True" w230 {
          tunnel: w235 -> [_ w246]
          tunnel: w234 -> [_ w245]
          tunnel: w232 -> [_ w244]
          frame False {
          }
          frame True {
            n102 = call-poly <vilib>:"DB Tools Execute Query.vi"("error in (no error)"=w245, "SQL query"=w244, "connection reference"=w246) -> ()  [unwired: 5 in, 2 out]
            "String" <- w244
          }
        }
        n103 = local write "Cmd."(w230) -> ()
      }
      frame "Get Image1" {
        # "EF01 FFFF FFFF 0100 0402 0100 08"
        n104 = flat-sequence {
          tunnel: w256 -> [w266]
          tunnel: w255 -> [w265]
          tunnel: [w262] -> w252
          tunnel: [w264] -> w250
          tunnel: [w263] -> w249
          tunnel: [w261] -> w248
          tunnel: w247 -> [w260]
          tunnel: [w268] -> w251
          tunnel: [w269] -> w253
          tunnel: [w270] -> w254
          tunnel: w250 -> [w270]
          tunnel: w249 -> [w269]
          tunnel: w248 -> [w268]
          frame #0 {
            n105 = call "Detect Finger.vi"("VISA Refnum in"=w266, "Cmd"="ï\u0001ÿÿÿÿ\u0001\u0000\u0004\u0002\u0001\u0000\b" ("write buffer"), "error in (no error)"=w265, "Buffer In"=w260) -> ("VISA Refnum out"=w264:refnum<visa-resource-name>, "Response"=w261:string, "Cmd Suceed?"=w262:bool, "error out"=w263:errorcluster)  [unwired: 6 in, 2 out]
          }
          frame #1 {
            n106 = disable-structure shown="Disabled" {
              frame Disabled {
                n107 = Wait (ms)(milliseconds to wait=u32 500) -> ()  [unwired: 1 out]
              }
              frame Enabled {
              }
            }
          }
        }
        n108 = Select(t=w259, s=w252, f=string[] []) -> (s? t:f=w258:string[])
      }
      frame "Get Image2" {
        # "EF01 FFFF FFFF 0100 0402 0200 09"
        n109 = flat-sequence {
          tunnel: w281 -> [w291]
          tunnel: w280 -> [w290]
          tunnel: [w287] -> w277
          tunnel: [w289] -> w275
          tunnel: [w288] -> w274
          tunnel: [w286] -> w273
          tunnel: w272 -> [w285]
          tunnel: [w293] -> w276
          tunnel: [w294] -> w278
          tunnel: [w295] -> w279
          tunnel: w275 -> [w295]
          tunnel: w274 -> [w294]
          tunnel: w273 -> [w293]
          frame #0 {
            n110 = call "Detect Finger.vi"("VISA Refnum in"=w291, "Cmd"="ï\u0001ÿÿÿÿ\u0001\u0000\u0004\u0002\u0002\u0000\t" ("write buffer"), "error in (no error)"=w290, "Buffer In"=w285) -> ("VISA Refnum out"=w289:refnum<visa-resource-name>, "Response"=w286:string, "Cmd Suceed?"=w287:bool, "error out"=w288:errorcluster)  [unwired: 6 in, 2 out]
          }
          frame #1 {
            n111 = disable-structure shown="Disabled" {
              frame Disabled {
                n112 = Wait (ms)(milliseconds to wait=u32 500) -> ()  [unwired: 1 out]
              }
              frame Enabled {
              }
            }
          }
        }
        n113 = Select(t=w284, s=w277, f=string[] []) -> (s? t:f=w283:string[])
      }
      frame "Merge Data" {
        n114 = call "Detect Finger.vi"("VISA Refnum in"=w304, "Cmd"="ï\u0001ÿÿÿÿ\u0001\u0000\u0003\u0005\u0000\t" ("write buffer"), "error in (no error)"=w303, "Buffer In"=w297) -> ("VISA Refnum out"=w302:refnum<visa-resource-name>, "Response"=w299:string, "Cmd Suceed?"=w300:bool, "error out"=w301:errorcluster)  [unwired: 6 in, 2 out]
        n115 = Select(t=w307, s=w300, f=string[] []) -> (s? t:f=w306:string[])
      }
      frame "Add Finger" {
        (unwired) "ï\u0001ÿÿÿÿ\u0001\u0000\u0006\u0006\u0002\u0000\u0000" ("write buffer")
        n116 = call <vilib>:"DB Tools Select Data.vi"("error in (no error)"=w330, "table"=w326, "connection reference"=w331) -> ("error out"=w327:errorcluster, "data"=w317:variant[][], "connection reference out"=w328:T6)  [unwired: 3 in]
        n117 = Variant To Data(type=string[][] [], Variant=w317) -> (data=w315:string[][])  [unwired: 1 in, 1 out]
        n118 = Index Array(array=w315, index (col)=0 ("disabled index (col)")) -> (element=w314:string[])  [unwired: 1 in]
        n119 = property on="Level" class="Enum (strict)"() -> ("RingText.Text"=w320:string)  [unwired: 2 in, 2 out]
        n120 = Decimal String To Number(string=w314) -> (number=w313:i32[])  [unwired: 2 in, 1 out]
        n121 = Get Date/Time In Seconds() -> (seconds since 1Jan1904=w321:timestamp)
        n122 = call "ID Generator.vi"("ID in"=w313) -> ("ID out"=w312:i32[])
        n123 = Index Array(array=w312) -> (element=w311:i32)  [unwired: 1 in]
        n124 = call <vilib>:"Trim Whitespace.vi"("string"="User Name") -> ("trimmed string"=w310:string)  [unwired: 1 in]
        n125 = call <vilib>:"Trim Whitespace.vi"("string"="Clock No.") -> ("trimmed string"=w309:string)  [unwired: 1 in]
        n126 = To Unsigned Word Integer(number=w311) -> (unsigned 16bit integer=w324:u16)
        n127 = Bundle By Name(cluster=T1 {"eRID"=0, "eRName"="", "eRClock"="", "eRDate"=timestamp(0 s since 1904-01-01), "eRLevel"="", "eRAdmin"="", "eRPassword"=""} ("Cluster"), "eRID"=w324, "eRName"=w310, "eRClock"=w309, "eRDate"=w321, "eRLevel"=w320) -> (w319:T1)
        n128 = call "Add Finger Cmd.vi"("ID NUMBER"=w324) -> ("Add Cmd"=w333:string)
        n129 = call "Detect Finger.vi"("VISA Refnum in"=w338, "Cmd"=w333, "error in (no error)"=w337, "Buffer In"=w332) -> ("VISA Refnum out"=w336:refnum<visa-resource-name>, "Response"=w334:string, "Cmd Suceed?"=w308:bool, "error out"=w335:errorcluster)  [unwired: 6 in, 2 out]
        n130 = To Variant(anything=w319) -> (Variant=w318:variant)
        n131 = case shown="True" w308 {
          tunnel: w328 -> [_ w345]
          tunnel: w327 -> [_ w344]
          tunnel: w326 -> [_ w343]
          tunnel: w318 -> [_ w342]
          frame False {
          }
          frame True {
            n132 = call <vilib>:"DB Tools Insert Data.vi"("data"=w342, "error in (no error)"=w344, "table"=w343, "connection reference"=w345) -> ()  [unwired: 6 in, 2 out]
          }
        }
        n133 = local write "Cmd."(w308) -> ()
        n134 = Select(t=w341, s=w308, f=string[] []) -> (s? t:f=w340:string[])
      }
      frame "Dummy" {
      }
      frame "Idle", Default {
        (unwired) "Search"
        n135 = disable-structure shown="Enabled" {
          disable-tunnel: 100 -> [w371 w456 _ _]
          disable-tunnel: w360 -> [w370 w455 _ _]
          disable-tunnel: [w369 w454 string[] ["Finger Presence1", "Get Image1", "Find Finger"] _] -> w359
          disable-tunnel: w358 -> [w368 w453 w632 _]
          disable-tunnel: w357 -> [w367 w452 w631 _]
          disable-tunnel: [w366 w451 w632 _] -> w356
          disable-tunnel: [w365 w450 w631 _] -> w355
          disable-tunnel: w353 -> [w364 w449 _ _]
          disable-tunnel: w352 -> [w363 w448 _ _]
          disable-tunnel: w351 -> [w362 w447 _ _]
          disable-tunnel: w350 -> [_ w446 _ _]
          frame Disabled {
            n136 = event shown="[6] \"Search\": Value Change" {
              selector: _ -> [_ _ _ _ _ _ _ _ _]
              dyn-events: _ -> [_ _ _ _ _ _ _ _ _]
              timeout: w371 -> [_ _ _ _ _ _ _ _ _]
              tunnel: w370 -> [w374 w384 w397 w403 w406 w408 _ w428 w437]
              tunnel: [w374 w384 w397 w403 w406 w418 string[] ["Finger Presence1", "Get Image1", "Find Finger"] w431 w440] -> w369
              tunnel: w368 -> [w373 w383 w396 w402 w405 w417 w427 w433 w442]
              tunnel: w367 -> [w372 w382 w395 w401 w404 w416 w426 w432 w441]
              tunnel: [w373 w383 w396 w402 w405 w417 w427 w433 w442] -> w366
              tunnel: [w372 w382 w395 w401 w404 w416 w426 w432 w441] -> w365
              tunnel: w364 -> [_ w380 w393 _ _ _ _ _ _]
              tunnel: w363 -> [_ w379 w392 _ _ _ _ _ _]
              tunnel: w362 -> [_ w378 _ _ _ _ _ _ _]
              event Timeout {
                n137 = event-data() -> ()  [unwired: 1 in, 1 out]
              }
              event "View All": Value Change {
                n138 = event-data() -> ("CtlRef"=w377:refnum<vi>)  [unwired: 1 in]
                n139 = call <vilib>:"DB Tools Select Data.vi"("error in (no error)"=w379, "table"=w378, "connection reference"=w380) -> ("data"=w381:variant[][])  [unwired: 3 in, 2 out]
                n140 = flat-sequence {
                  tunnel: w381 -> [w387]
                  tunnel: [errorcluster {"status"=FALSE, "code"=0, "source"=""} ("error in (no error)")] -> w376
                  frame #0 {
                    n141 = call "1775E_User List.vi"("Log?"=TRUE, "data"=w387) -> ()  [unwired: 10 in]
                  }
                }
                n142 = property class="Bool (strict)"(reference=w377, error in=w376, "Value"=FALSE) -> ()  [unwired: 2 out]
              }
              event "View Log": Value Change {
                n143 = event-data() -> ("CtlRef"=w391:refnum<vi>)  [unwired: 1 in]
                n144 = call <vilib>:"DB Tools Select Data.vi"("error in (no error)"=w392, "table"="UserLogin", "connection reference"=w393) -> ("data"=w394:variant[][])  [unwired: 3 in, 2 out]
                n145 = flat-sequence {
                  tunnel: w394 -> [w400]
                  tunnel: [errorcluster {"status"=FALSE, "code"=0, "source"=""} ("error in (no error)")] -> w390
                  frame #0 {
                    n146 = call "1775E_User List.vi"("Log?"=FALSE, "data"=w400) -> ()  [unwired: 10 in]
                  }
                }
                n147 = property class="Bool (strict)"(reference=w391, error in=w390, "Value"=FALSE) -> ()  [unwired: 2 out]
              }
              event "Super User": Value Change {
                n148 = event-data() -> ()  [unwired: 1 in, 1 out]
              }
              event "Stop": Value Change {
                n149 = event-data() -> ()  [unwired: 1 in, 1 out]
              }
              event "Enroll": Value Change {
                n150 = event-data() -> ()  [unwired: 1 in, 1 out]
                n151 = local read "Clock No."() -> (w414:string)
                n152 = local read "User Name"() -> (w415:string)
                n153 = call <vilib>:"Trim Whitespace.vi"("string"=w414) -> ("trimmed string"=w413:string)  [unwired: 1 in]
                n154 = call <vilib>:"Trim Whitespace.vi"("string"=w415) -> ("trimmed string"=w412:string)  [unwired: 1 in]
                n155 = Empty String/Path?(string/path=w413) -> (empty?=w411:bool)
                n156 = Empty String/Path?(string/path=w412) -> (empty?=w410:bool)
                n157 = Compound Arithmetic op=OR(w411, w410) -> (w409:bool)
                n158 = case shown="True" w409 {
                  selector: w409 -> [w419 _]
                  tunnel: [string[] ["Finger Presence1", "Get Image1", "Remove Finger", "Finger Presence2", "Get Image2", "Merge Data", "Add Finger"] w422] -> w418
                  tunnel: w408 -> [_ w422]
                  tunnel: [w419 _] -> w407
                  frame False {
                  }
                  frame True {
                    n159 = call <userlib>:"Warning .vi"("Warning in"="Empty User Name or Clock No.") -> ()  [unwired: 15 in]
                  }
                }
                n160 = local write "Enroll"(w407) -> ()
              }
              event "Search": Value Change {
                w423 = "" ("User Name")
                n161 = event-data() -> ()  [unwired: 1 in, 1 out]
                n162 = local write "User Name"(w423) -> ()
                n163 = local write "Clock No."(w423) -> ()
                n164 = local write "ID Number"(i16 -1 ("ID")) -> ()
              }
              event "Delete All": Value Change {
                n165 = event-data() -> ()  [unwired: 1 in, 1 out]
                n166 = call <userlib>:"Warning With option(W).vi"("Warning in"="Are you sure you want to Delete all Users?") -> ("Cancel ?"=w429:bool)  [unwired: 13 in, 1 out]
                n167 = case shown="False" w429 {
                  tunnel: [string[] ["Delete All"] w435] -> w431
                  tunnel: w428 -> [_ w435]
                  frame False {
                  }
                  frame True {
                  }
                }
              }
              event "Delete": Value Change {
                (unwired) "Search"
                n168 = event-data() -> ()  [unwired: 1 in, 1 out]
                n169 = call <userlib>:"Warning With option(W).vi"("Warning in"="Are you sure you want to Delete this User ID?") -> ("Cancel ?"=w438:bool)  [unwired: 13 in, 1 out]
                n170 = case shown="False" w438 {
                  selector: w438 -> [w443 _]
                  tunnel: [string[] ["Delete ID"] w445] -> w440
                  tunnel: w437 -> [_ w445]
                  tunnel: [w443 _] -> w436
                  frame False {
                  }
                  frame True {
                  }
                }
                n171 = local write "Delete"(w436) -> ()
              }
            }
          }
          frame Enabled {
            n172 = event shown="[7] \"Password\": Value Change" {
              selector: _ -> [_ _ _ _ _ _ _ _ _ _ _]
              dyn-events: _ -> [_ _ _ _ _ _ _ _ _ _ _]
              timeout: w456 -> [_ _ _ _ _ _ _ _ _ _ _]
              tunnel: w455 -> [w458 w481 w494 w500 w503 w505 _ w554 w608 w611 w620]
              tunnel: [w459 w481 w494 w500 w503 w515 w520 w554 w608 w614 w623] -> w454
              tunnel: w453 -> [w462 w480 w493 w499 w502 w514 w527 w556 w610 w616 w625]
              tunnel: w452 -> [w461 w479 w492 w498 w501 w513 w526 w555 w609 w615 w624]
              tunnel: [w462 w480 w493 w499 w502 w514 w527 w556 w610 w616 w625] -> w451
              tunnel: [w461 w479 w492 w498 w501 w513 w526 w555 w609 w615 w624] -> w450
              tunnel: w449 -> [_ w477 w490 _ _ _ _ w553 w607 _ _]
              tunnel: w448 -> [_ w476 w489 _ _ _ _ w552 w606 _ _]
              tunnel: w447 -> [_ w475 _ _ _ _ _ _ _ _ _]
              tunnel: w446 -> [_ _ _ _ _ _ _ w530 _ _ _]
              event Timeout {
                n173 = event-data() -> ()  [unwired: 1 in, 1 out]
                n174 = property on="Search" class="Bool (strict)"() -> ("DisabledEnum"=w460:T4, "Value"=w457:bool)  [unwired: 2 in, 2 out]
                n175 = disable-structure shown="Enabled" {
                  disable-tunnel: w460 -> [w465 _ _]
                  disable-tunnel: [w464 w469 _] -> w459
                  disable-tunnel: w458 -> [w463 _ _]
                  disable-tunnel: w457 -> [_ w468 _]
                  frame Disabled {
                    n176 = case shown="\"Disabled\", Default" w465 {
                      tunnel: [w466 string[] ["Finger Presence1", "Get Image1", "Find Finger"]] -> w464
                      tunnel: w463 -> [w466 _]
                      frame "Enabled" {
                      }
                      frame "Disabled", Default {
                      }
                    }
                  }
                  frame Enabled {
                    n177 = case shown="True" w468 {
                      tunnel: [string[] ["Finger Presence1", "Get Image1", "Find Finger"] string[] []] -> w469
                      frame False {
                      }
                      frame True {
                      }
                    }
                  }
                  frame Disabled {
                  }
                }
              }
              event "View All": Value Change {
                n178 = event-data() -> ("CtlRef"=w474:refnum<vi>)  [unwired: 1 in]
                n179 = call <vilib>:"DB Tools Select Data.vi"("error in (no error)"=w476, "table"=w475, "connection reference"=w477) -> ("data"=w478:variant[][])  [unwired: 3 in, 2 out]
                n180 = flat-sequence {
                  tunnel: w478 -> [w484]
                  tunnel: [errorcluster {"status"=FALSE, "code"=0, "source"=""} ("error in (no error)")] -> w473
                  frame #0 {
                    n181 = call "1775E_User List.vi"("Log?"=TRUE, "data"=w484) -> ()  [unwired: 10 in]
                  }
                }
                n182 = property class="Bool (strict)"(reference=w474, error in=w473, "Value"=FALSE) -> ()  [unwired: 2 out]
              }
              event "View Log": Value Change {
                n183 = event-data() -> ("CtlRef"=w488:refnum<vi>)  [unwired: 1 in]
                n184 = call <vilib>:"DB Tools Select Data.vi"("error in (no error)"=w489, "table"="UserLogin", "connection reference"=w490) -> ("data"=w491:variant[][])  [unwired: 3 in, 2 out]
                n185 = flat-sequence {
                  tunnel: w491 -> [w497]
                  tunnel: [errorcluster {"status"=FALSE, "code"=0, "source"=""} ("error in (no error)")] -> w487
                  frame #0 {
                    n186 = call "1775E_User List.vi"("Log?"=FALSE, "data"=w497) -> ()  [unwired: 10 in]
                  }
                }
                n187 = property class="Bool (strict)"(reference=w488, error in=w487, "Value"=FALSE) -> ()  [unwired: 2 out]
              }
              event "Super User": Value Change {
                n188 = event-data() -> ()  [unwired: 1 in, 1 out]
              }
              event "Stop": Value Change {
                n189 = event-data() -> ()  [unwired: 1 in, 1 out]
              }
              event "Enroll": Value Change {
                n190 = event-data() -> ()  [unwired: 1 in, 1 out]
                n191 = local read "Clock No."() -> (w511:string)
                n192 = local read "User Name"() -> (w512:string)
                n193 = call <vilib>:"Trim Whitespace.vi"("string"=w511) -> ("trimmed string"=w510:string)  [unwired: 1 in]
                n194 = call <vilib>:"Trim Whitespace.vi"("string"=w512) -> ("trimmed string"=w509:string)  [unwired: 1 in]
                n195 = Empty String/Path?(string/path=w510) -> (empty?=w508:bool)
                n196 = Empty String/Path?(string/path=w509) -> (empty?=w507:bool)
                n197 = Compound Arithmetic op=OR(w508, w507) -> (w506:bool)
                n198 = case shown="True" w506 {
                  selector: w506 -> [w516 _]
                  tunnel: [string[] ["Finger Presence1", "Get Image1", "Remove Finger", "Finger Presence2", "Get Image2", "Merge Data", "Add Finger"] w519] -> w515
                  tunnel: w505 -> [_ w519]
                  tunnel: [w516 _] -> w504
                  frame False {
                  }
                  frame True {
                    n199 = call <userlib>:"Warning .vi"("Warning in"="Empty User Name or Clock No.") -> ()  [unwired: 15 in]
                  }
                }
                n200 = local write "Enroll"(w504) -> ()
              }
              event "Search": Value Change {
                w523 = "" ("User Name")
                (unwired) string[] ["Finger Presence1", "Get Image1", "Find Finger"]
                n201 = event-data() -> ("NewVal"=w521:bool)  [unwired: 1 in]
                n202 = local write "Password"(w523) -> ()
                n203 = local write "Clock No."(w523) -> ()
                n204 = case shown="False" w521 {
                  tunnel: [string[] ["Finger Presence1", "Get Image1", "Find Finger"] string[] []] -> w520
                  frame False {
                  }
                  frame True {
                  }
                }
                n205 = local write "ID Number"(i16 -1 ("ID")) -> ()
                n206 = property on="Ok" class="Bool (strict)"("DisabledEnum"=T4."Disabled and Grayed Out" ("Disabled")) -> ()  [unwired: 2 in, 2 out]
                n207 = property on="Search" class="Bool (strict)"("DisabledEnum"=T4."Enabled" ("Disabled")) -> ()  [unwired: 2 in, 2 out]
              }
              event "Password": Value Change {
                n208 = event-data() -> ("NewVal"=w532:string)  [unwired: 1 in]
                n209 = local read "Clock No."() -> (w549:string)
                n210 = local read "User Name"() -> (w550:string)
                n211 = Format Into String(format string="SELECT *  FROM [dbo].[User_Management] Where eRName = '%s' and eRClock = '%s'" ("SQL query"), w550, w549) -> (resulting string=w544:string)  [unwired: 2 in, 1 out]
                n212 = call-poly <vilib>:"DB Tools Execute Query.vi"("error in (no error)"=w552, "SQL query"=w544, "connection reference"=w553) -> ("error out"=w543:errorcluster, "recordset reference"=w546:T9)  [unwired: 5 in]
                n213 = call-poly <vilib>:"DB Tools Fetch Recordset Data.vi"("error in (no error)"=w543, "recordset reference"=w546) -> ("error out"=w548:errorcluster, "recordset data"=w536:variant[][], "recordset reference out"=w547:T9)  [unwired: 3 in]
                n214 = Index Array(array=w536, index (row)=0 ("disabled index (col)")) -> (element=w542:variant[])  [unwired: 1 in]
                n215 = call-poly <vilib>:"DB Tools Free Object.vi"("error in (no error)"=w548, "recordset reference"=w547) -> ("error out"=w534:errorcluster, "connection reference"=w535:T6)  [unwired: 8 in]
                n216 = Variant To Data(type=string[] [], Variant=w542) -> (data=w540:string[])  [unwired: 1 in, 1 out]
                n217 = Index Array(array=w540, index=6) -> (element=w538:string)
                n218 = call <vilib>:"Trim Whitespace.vi"("string"=w538) -> ("trimmed string"=w537:string)  [unwired: 1 in]
                n219 = call "Password.vi"("Password In"=w537) -> ("Password out"=w533:string)
                n220 = Equal?(x=w532, y=w533) -> (x = y?=w531:bool)
                n221 = case shown="True" w531 {
                  tunnel: w536 -> [_ w563]
                  tunnel: w535 -> [_ w562]
                  tunnel: w534 -> [_ w561]
                  tunnel: w530 -> [_ w558]
                  frame False {
                    n222 = local write "Response"("Incorrect Password" ("Response")) -> ()
                  }
                  frame True {
                    n223 = Index Array(array=w563, index (row)=0 ("disabled index (col)")) -> (element=w584:variant[])  [unwired: 1 in]
                    n224 = call <userlib>:"Array of VData to VCluster__ogtk.vi"("Array"=w584) -> ("VCluster"=w586:variant)  [unwired: 9 in, 1 out]
                    n225 = Variant To Data(type=string[] [], Variant=w584) -> (data=w582:string[])  [unwired: 1 in, 1 out]
                    n226 = Variant To Data(type=T1 {"eRID"=0, "eRName"="", "eRClock"="", "eRDate"=timestamp(0 s since 1904-01-01), "eRLevel"="", "eRAdmin"="", "eRPassword"=""} ("Cluster"), Variant=w586) -> (data=w580:T1)  [unwired: 1 in, 1 out]
                    n227 = Index Array(array=w582) -> (element=w581:string)  [unwired: 1 in]
                    n228 = Decimal String To Number(string=w581) -> (number=w572:i32)  [unwired: 2 in, 1 out]
                    n229 = Bundle By Name(cluster=w580, "eRID"=w572) -> (w588:T1)
                    n230 = local write "Response"("Login Success." ("Response")) -> ()
                    n231 = Unbundle By Name(w580) -> ("eRLevel"=w579:string, "eRName"=w577:string, "eRClock"=w576:string)
                    n232 = local write "Ok"(TRUE ("Ok")) -> ()
                    n233 = property on="Level" class="Enum (strict)"() -> ("Strings []"=w575:string[])  [unwired: 2 in, 2 out]
                    n234 = local write "data"(w588) -> ()
                    n235 = call <vilib>:"Trim Whitespace.vi"("string"=w579) -> ("trimmed string"=w569:string)  [unwired: 1 in]
                    n236 = call <vilib>:"Trim Whitespace.vi"("string"=w577) -> ("trimmed string"=w571:string)  [unwired: 1 in]
                    n237 = call <vilib>:"Trim Whitespace.vi"("string"=w576) -> ("trimmed string"=w570:string)  [unwired: 1 in]
                    n238 = Search 1D Array(1D array=w575, element=w569) -> (index of element=w578:i32)  [unwired: 1 in]
                    n239 = local write "User Name"(w571) -> ()
                    n240 = local write "Clock No."(w570) -> ()
                    n241 = local write "Level"(w578) -> ()
                    n242 = Get Date/Time In Seconds() -> (seconds since 1Jan1904=w568:timestamp)
                    n243 = Bundle By Name(cluster=T8 {"eRID"=0, "eRName"="", "eRClock"="", "eRDate"=timestamp(0 s since 1904-01-01), "eRLevel"="", "eRAdmin"="", "eRPassword"="", "eRPurpose"=""} ("Cluster"), "eRID"=w572, "eRName"=w571, "eRClock"=w570, "eRDate"=w568, "eRLevel"=w569, "eRAdmin"="", "eRPassword"="Password", "eRPurpose"=w558) -> (w567:T8)
                    n244 = To Variant(anything=w567) -> (Variant=w566:variant)
                    n245 = call <vilib>:"DB Tools Insert Data.vi"("data"=w566, "error in (no error)"=w561, "table"="UserLogin", "connection reference"=w562) -> ()  [unwired: 6 in, 2 out]
                  }
                }
              }
              event "User Name": Value Change {
                n246 = event-data() -> ("NewVal"=w595:string)  [unwired: 1 in]
                n247 = Format Into String(format string="SELECT [eRClock],[eRLevel] FROM [dbo].[User_Management] where [eRName] = '%s' order by [eRClock] asc" ("Response"), w595) -> (resulting string=w601:string)  [unwired: 2 in, 1 out]
                n248 = call-poly <vilib>:"DB Tools Execute Query.vi"("error in (no error)"=w606, "SQL query"=w601, "connection reference"=w607) -> ("error out"=w600:errorcluster, "recordset reference"=w603:T9)  [unwired: 5 in]
                n249 = call-poly <vilib>:"DB Tools Fetch Recordset Data.vi"("error in (no error)"=w600, "recordset reference"=w603) -> ("error out"=w605:errorcluster, "recordset data"=w597:variant[][], "recordset reference out"=w604:T9)  [unwired: 3 in]
                n250 = Index Array(array=w597, index (row)=0 ("disabled index (col)")) -> (element=w599:variant[])  [unwired: 1 in]
                n251 = call-poly <vilib>:"DB Tools Free Object.vi"("error in (no error)"=w605, "recordset reference"=w604) -> ()  [unwired: 8 in, 2 out]
                n252 = Variant To Data(type=string[] [], Variant=w599) -> (data=w593:string[])  [unwired: 1 in, 1 out]
                n253 = Index Array(array=w593) -> (element #1=w594:string, element #2=w589:string)  [unwired: 2 in]
                n254 = property on="Clock No." class="CmbBox"("Strings[]"=w593, "Value"=w594) -> ()  [unwired: 2 in, 2 out]
                n255 = call <vilib>:"Trim Whitespace.vi"("string"=w589) -> ("trimmed string"=w591:string)  [unwired: 1 in]
                n256 = property on="Level" class="Enum (strict)"() -> ("Strings []"=w592:string[])  [unwired: 2 in, 2 out]
                n257 = Search 1D Array(1D array=w592, element=w591) -> (index of element=w590:i32)  [unwired: 1 in]
                n258 = local write "Level"(w590) -> ()
              }
              event "Delete All": Value Change {
                n259 = event-data() -> ()  [unwired: 1 in, 1 out]
                n260 = call <userlib>:"Warning With option(W).vi"("Warning in"="Are you sure you want to Delete all Users?") -> ("Cancel ?"=w612:bool)  [unwired: 13 in, 1 out]
                n261 = case shown="False" w612 {
                  tunnel: [string[] ["Delete All"] w618] -> w614
                  tunnel: w611 -> [_ w618]
                  frame False {
                  }
                  frame True {
                  }
                }
              }
              event "Delete": Value Change {
                (unwired) "Search"
                n262 = event-data() -> ()  [unwired: 1 in, 1 out]
                n263 = call <userlib>:"Warning With option(W).vi"("Warning in"="Are you sure you want to Delete this User ID?") -> ("Cancel ?"=w621:bool)  [unwired: 13 in, 1 out]
                n264 = case shown="False" w621 {
                  selector: w621 -> [w626 _]
                  tunnel: [string[] ["Delete ID"] w628] -> w623
                  tunnel: w620 -> [_ w628]
                  tunnel: [w626 _] -> w619
                  frame False {
                  }
                  frame True {
                  }
                }
                n265 = local write "Delete"(w619) -> ()
              }
            }
          }
          frame Disabled {
            w629 = "" ("User Name")
            n266 = local write "User Name"(w629) -> ()
            n267 = local write "Clock No."(w629) -> ()
            n268 = local write "ID Number"(i16 -1 ("ID")) -> ()
          }
          frame Disabled {
          }
        }
      }
      frame "Init" {
        n269 = invoke class="VI" method="Default Vals.Reinit All"() -> (error out=w639:errorcluster)  [unwired: 3 in, 2 out]
        n270 = stacked-sequence {
          tunnel: [w652 _] -> w645
          tunnel: w644 -> [_ w690]
          tunnel: [_ w689] -> w643
          tunnel: w642 -> [_ w688]
          tunnel: w641 -> [_ w686]
          tunnel: [_ w685] -> w640
          tunnel: w639 -> [_ _]
          tunnel: [_ w676] -> w637
          tunnel: w636 -> [w666 _]
          frame #0 {
            w654 = 0 ("index (row)")
            w652 = "Enter User Details" ("Response")
            (unwired) "Wait for Finger Print Connection." ("Response")
            n271 = call-poly <vilib>:"DB Tools Execute Query.vi"("SQL query"="SELECT [eRName] FROM [dbo].[User_Management] order by [eRName] asc" ("Response"), "connection reference"=w666) -> ("error out"=w670:errorcluster, "recordset reference"=w671:T9)  [unwired: 6 in]
            n272 = call-poly <vilib>:"DB Tools Fetch Recordset Data.vi"("error in (no error)"=w670, "recordset reference"=w671) -> ("error out"=w673:errorcluster, "recordset data"=w668:variant[][], "recordset reference out"=w672:T9)  [unwired: 3 in]
            n273 = Index Array(array=w668, index (col)=0 ("disabled index (col)")) -> (element=w669:variant[])  [unwired: 1 in]
            n274 = call-poly <vilib>:"DB Tools Free Object.vi"("error in (no error)"=w673, "recordset reference"=w672) -> ("error out"=w659:errorcluster, "connection reference"=w660:T6)  [unwired: 8 in]
            n275 = Variant To Data(type=string[] [], Variant=w669) -> (data=w651:string[])  [unwired: 1 in, 1 out]
            n276 = call-poly <vilib>:"DB Tools Execute Query.vi"("error in (no error)"=w659, "SQL query"="SELECT TOP 1 [eRName] FROM [CELL10].[dbo].[UserLogin] ORDER BY eRDate DESC" ("Response"), "connection reference"=w660) -> ("error out"=w658:errorcluster, "recordset reference"=w662:T9)  [unwired: 5 in]
            n277 = call-poly <vilib>:"DB Tools Fetch Recordset Data.vi"("error in (no error)"=w658, "recordset reference"=w662) -> ("error out"=w657:errorcluster, "recordset data"=w655:variant[][], "recordset reference out"=w661:T9)  [unwired: 3 in]
            n278 = call-poly <vilib>:"DB Tools Free Object.vi"("error in (no error)"=w657, "recordset reference"=w661) -> ()  [unwired: 8 in, 2 out]
            n279 = Index Array(array=w655, index (row)=w654, index (col)=w654) -> (element=w653:variant)
            n280 = Variant To Data(type=w652, Variant=w653) -> (data=w650:string)  [unwired: 1 in, 1 out]
            n281 = local write "Response"(w652) -> ()
            n282 = Search 1D Array(1D array=w651, element=w650) -> (index of element=w649:i32)  [unwired: 1 in]
            n283 = Max & Min(x=0, y=w649) -> (max(x,y)=w647:i32)  [unwired: 1 out]
            n284 = Index Array(array=w651, index=w647) -> (element=w663:string)
            n285 = property on="User Name" class="CmbBox"("Strings[]"=w651, "Val(Sgnl)"=w663) -> ()  [unwired: 2 in, 2 out]
          }
          frame #1 {
            w679 = "" ("User Name")
            n286 = property on="Level" class="Enum (strict)"("Disabled Items []"=i32[] [4]) -> ()  [unwired: 2 in, 2 out]
            n287 = call "Detect Finger.vi"("VISA Refnum in"=w690, "Cmd"="ï\u0001ÿÿÿÿ\u0001\u0000\u0003\u0016\u0000\u001a", "error in (no error)"=w686, "Buffer In"=w688) -> ("VISA Refnum out"=w689:refnum<visa-resource-name>, "Cmd Suceed?"=→"Cmd Suceed?":bool, "Buffer Out"=w687:string, "error out"=w685:errorcluster)  [unwired: 6 in, 2 out]
            n288 = local write "ID Number"(i16 -1 ("ID")) -> ()
            n289 = property on="Search" class="Bool (strict)"("DisabledEnum"=T4."Enabled" ("Disabled")) -> ()  [unwired: 2 in, 2 out]
            n290 = local write "Stop"(FALSE ("Stop")) -> ()
            n291 = property on="Ok" class="Bool (strict)"("DisabledEnum"=T4."Disabled and Grayed Out" ("Disabled")) -> (error out=w676:errorcluster)  [unwired: 2 in, 1 out]
            n292 = call "Get Device Info.vi"("Read Data"=w687) -> ("Device Info"=→"Device Info":string)
            n293 = local write "Clock No."(w679) -> ()
            n294 = local write "Password"(w679) -> ()
            n295 = disable-structure shown="Disabled" {
              frame Disabled {
                n296 = property on="Search" class="Bool (strict)"("Val(Sgnl)"=TRUE ("Value (Signaling)")) -> ()  [unwired: 2 in, 2 out]
              }
              frame Enabled {
              }
            }
            "Cmd." <- FALSE ("Cmd.")
          }
        }
        n297 = property on="Hide" class="Bool"(error in=w637, "Visible"=FALSE) -> (error out=w634:errorcluster)  [unwired: 1 in, 1 out]
        n298 = property on="Password" class="Str"(error in=w634, "Key Focus"=TRUE) -> ()  [unwired: 1 in, 2 out]
      }
    }
    n299 = Wait (ms)(milliseconds to wait=u32 100) -> ()  [unwired: 1 out]
    n300 = Compound Arithmetic op=OR(w82, "Stop", "Cancel", "Ok") -> (w84:bool)
    "Numeric" <- w73
    "Array" <- w93
  }
  n301 = Not(x=w8) -> (.not. x?=→"Cancel ?":bool)
  n302 = VISA Close(VISA resource name=w14, error in (no error)=w13) -> (error out=w12:errorcluster)
  n303 = call <vilib>:"Clear Errors.vi"("error in (no error)"=w12) -> ()  [unwired: 5 in, 2 out]
